vi "Auto_New.vi"() -> ()   [LabVIEW 2017]
uses:
  Control/Saurabh/prosucer_consumer_enum1.ctl
  Control/OUTPUT Cluster Indicator.ctl
  <vilib>/Utility/error.llb/DialogType.ctl
  <vilib>/addons/database/Connection.llb/DB Tools Open Connec (String).vi
  Global/DATA LOG.vi
  Global/Global 1.vi
  <vilib>/addons/database/NI_Database_API.lvlib
panel:
  out "SHIFT":string
  in  "BARCODE RECIPE":string(combo)
  out "PLC COM.":bool
  out "SHIFT_DATA":string[](array[string])
  out "stop":bool
  out "error out 2":errorcluster
  out "Shift 4":i32
  out "Time Stamp Out":timestamp[](array[timestamp]) format="%<%X>T"
  out "Time Stamp Out 4":timestamp[](array[timestamp]) format="%<%X>T"
  out "Shift_change":bool
  out "appended array":string[][](array[string])
  out "SHIFT_DATA 2":string[](array[string])
  in  "error in (no error)":errorcluster
  in  "Tab Control":T1(tab)
  out "OP 50":bool
  out "OP 40":bool
  out "OP 30":bool
  out "OP - 50":T2 {"RH Motor Screw" format="%#.2g N-m"; "LH Motor Screw" format="%#.2g N-m"; "Nut Torque" format="%#.2g N-m"}
  out "OP - 40":T3 {"Stack Load" format="%.2f kg"; "Dispalcement" format="%#.2g mm"; "LH Screw" format="%#.2g N-m"; "RH Screw" format="%#.2g N-m"}
  out "OP - 30":T4 {"Shaft Press Load" format="%#.2g kg"; "Displacement" format="%#.2g mm"}
  in  "stop 2":bool
  out "OP - 10":T5 {"Leak Rate" format="%#.2g SCCM"}
  in  "SIMULATE INPUT":bool[](array[boolean])=[FALSE, FALSE, FALSE, FALSE]
  out "OP - 20":T6 {"Top Load" format="%#.2g kg"; "Top Displace" format="%#.2g mm"; "Bottom Load" format="%#.2g kg"; "Bottom Displace" format="%#.2g mm"}
  out "OP 10 & 20":bool
  out "OP - 60":T7 {"Screw 6" format="%#.2g N-m"; "Screw 5" format="%#.2g N-m"; "Screw 4" format="%#.2g N-m"; "Screw 3" format="%#.2g N-m"; "Screw 2" format="%#.2g N-m"; "Screw 1" format="%#.2g N-m"}
  out "OP - 70":T8 {"Full Open" format="%#.4g V"; "Full Close" format="%#.4g V"}
  out "OP - 110":T9
  out "OP - 80":T10 {"Plug Press Load" format="%#.2f kg"}
  out "OP - 90":T11 {"Steam Leak" format="%#_g sccm"; "Seat Leak" format="%#_g LPM"}
  out "OP - 100":T12 {"Response Time REV" format="%#_g msec"; "Response time FWD" format="%#_g msec"; "Motor Full Open" format="%#.2f V"; "Motor Start Back" format="%#.2f V"; "Motor Full Close" format="%#.2f V"; "Motor Start Of Close" format="%#.2f V"; "Motor Peak" format="%#.2f A"; "Sensor O/P Full Close" format="%#.2f V"; "Sensor O/P Start Of Close" format="%#.2f V"; "Sensor O/P Open" format="%#.2f V"}
  out "OP 60":bool
  out "OP 70 & 80":bool
  out "OP 90 -100":bool
  out "OP 110":bool
  out "OP110 STATUS":dbl[](array[numeric])
  out "SCAN OP110":string[](array[string])
  out "OP100 STATUS":dbl[](array[numeric])
  out "SCAN OP100":string[](array[string])
  out "OP50 STATUS":dbl[](array[numeric])
  out "SCAN OP50":string[](array[string])
  out "OP90 STATUS":dbl[](array[numeric])
  out "SCAN OP90":string[](array[string])
  out "OP80 STATUS":dbl[](array[numeric])
  out "SCAN OP80":string[](array[string])
  out "OP70 STATUS":dbl[](array[numeric])
  out "SCAN OP70":string[](array[string])
  out "OP60 STATUS":dbl[](array[numeric])
  out "SCAN OP60":string[](array[string])
  out "OP40 STATUS":dbl[](array[numeric])
  out "SCAN OP40":string[](array[string])
  out "OP30 STATUS":dbl[](array[numeric])
  out "SCAN OP30":string[](array[string])
  out "OP20 STATUS":dbl[](array[numeric])
  out "SCAN OP20":string[](array[string])
  out "OP10 STATUS":dbl[](array[numeric])
  out "SCAN OP10":string[](array[string])
  out "resulting string":string
  out "PLC1 error":errorcluster
  out "PLC2 error":errorcluster
  out "PLC3 error":errorcluster
  out "PLC4 error":errorcluster
  out "PLC5 error":errorcluster
  out "PLC6 error":errorcluster
  out "PLC7 error":errorcluster
  out "PLC8 error":errorcluster
  # "Op10 20\nOp30\nOp 40\nOp50\nOp60\nOp70-80\nOp 90-100-110"
  # "SENSOR MIN VLTG"
  # "OP - 50"
  # "OP - 40"
  # "OP - 30"
  # "OP - 10"
  # "OP - 20"
  # "OP - 60"
  # "OP - 70"
  # "OP - 110"
  # "OP - 80"
  # "OP - 90"
  # "OP - 100"
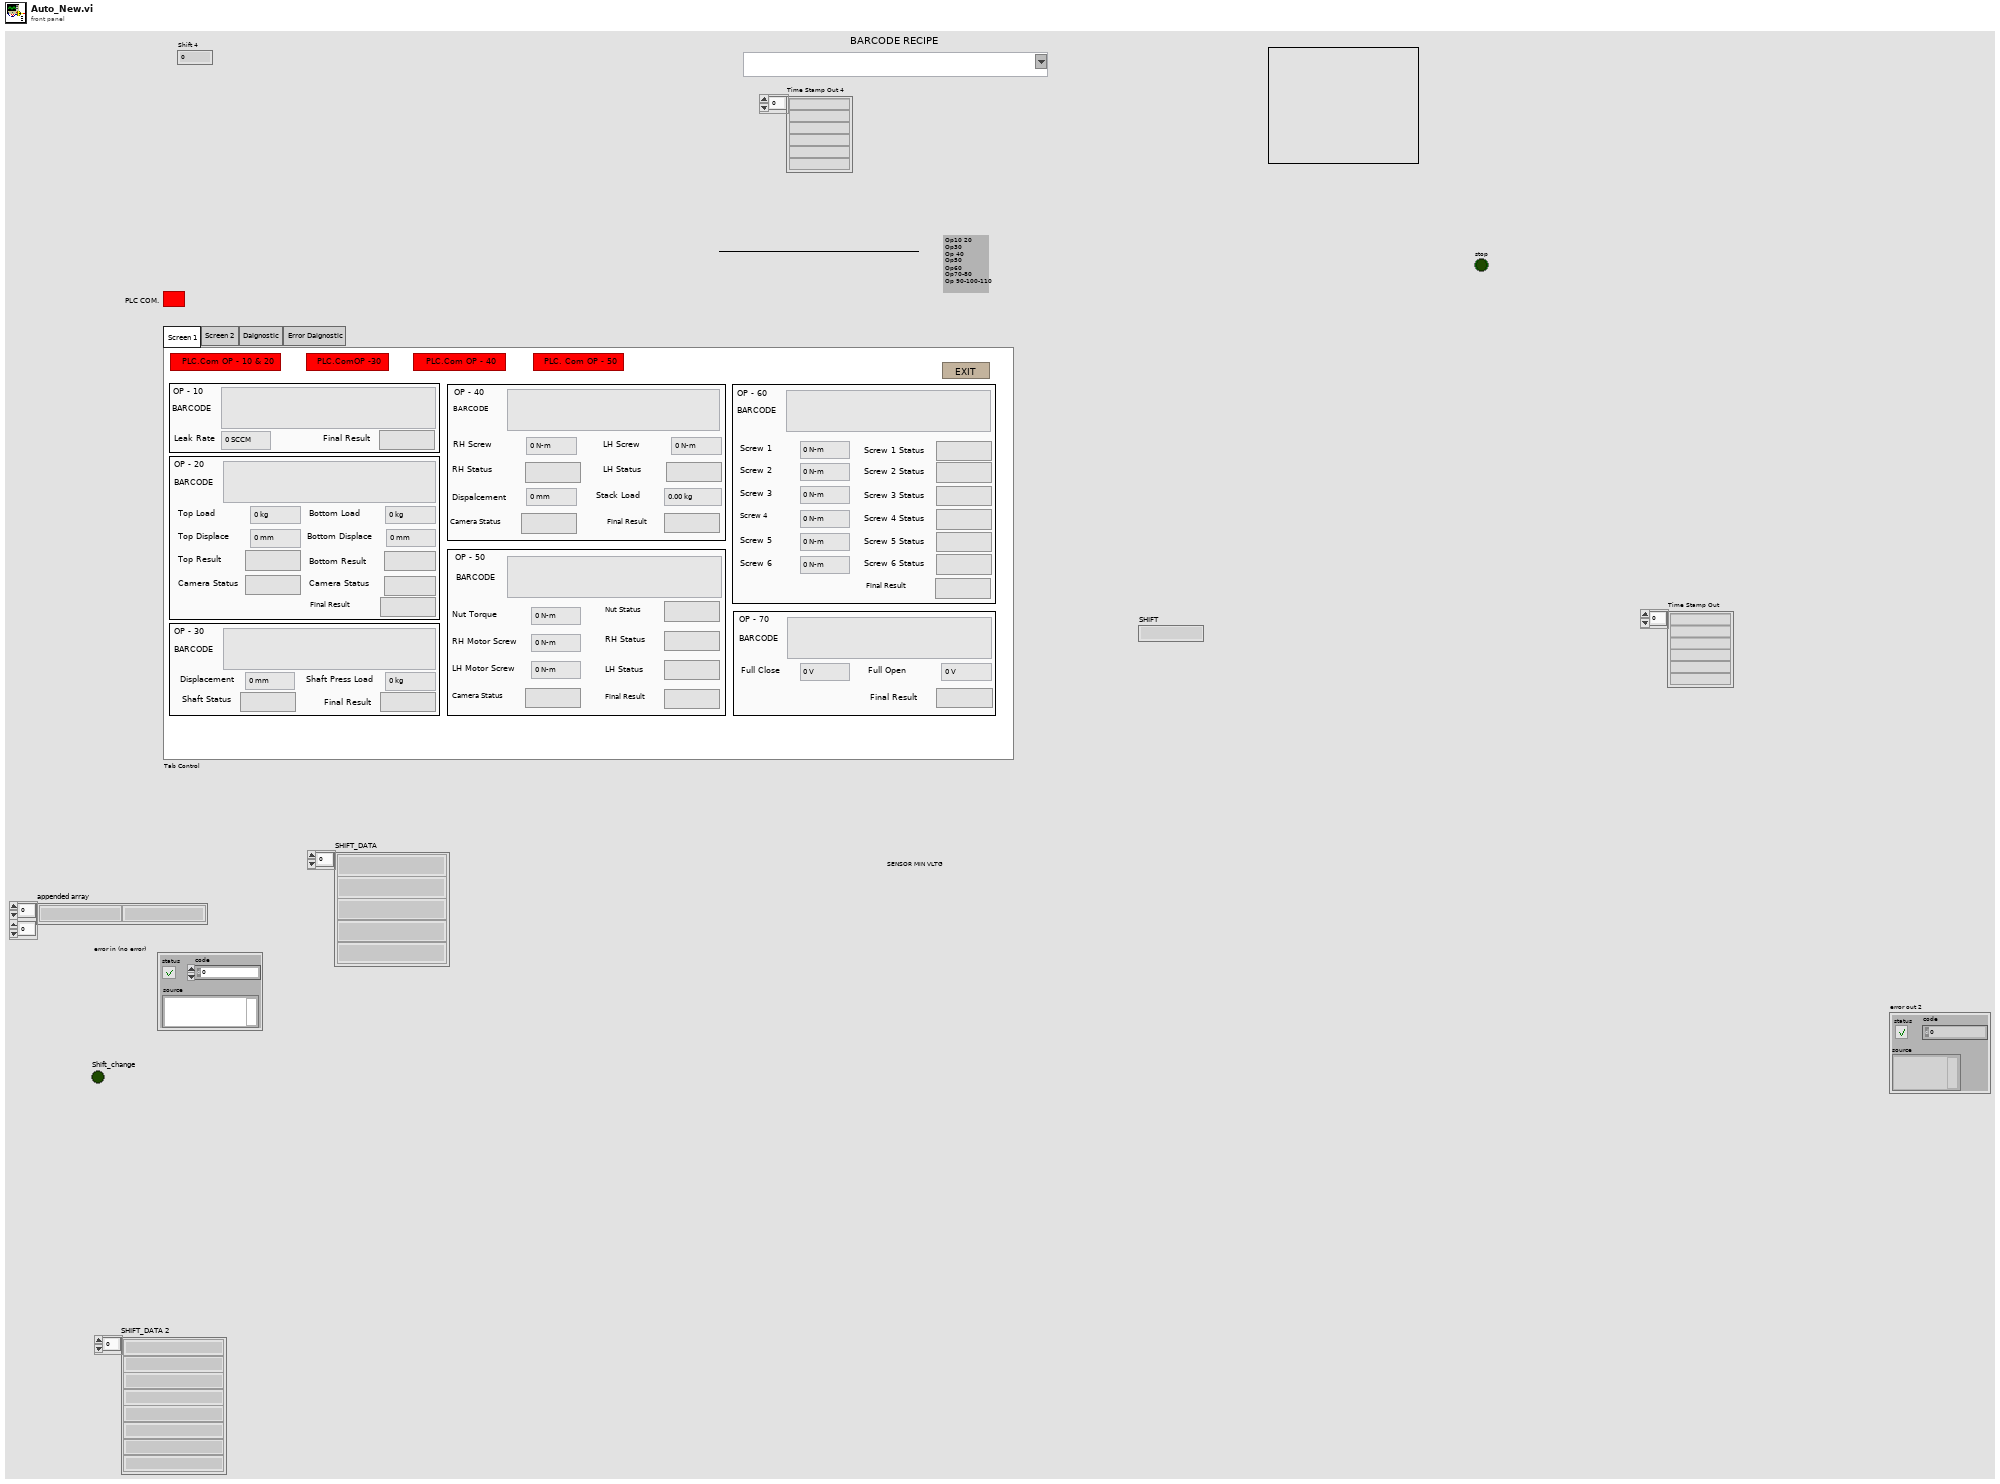
[diagram p1: front panel]
types:
  T1 = enum32{"Screen 1", "Screen 2", "Daignostic", "Error Daignostic"}
  T2 = cluster{"BARCODE":string, "Nut Torque":dbl, "LH Motor Screw":dbl, "LH Status":bool, "RH Status":bool, "RH Motor Screw":dbl, "Final Result":bool, "Nut Status":bool, "Camera Status":bool}
  T3 = cluster{"BARCODE":string, "RH Screw":dbl, "LH Screw ":dbl, "RH Status":bool, "LH Status":bool, "Dispalcement ":dbl, "Stack Load ":dbl, "Final Result":bool, "Camera Status":bool}
  T4 = cluster{"BARCODE":string, "Displacement":dbl, "Shaft Press Load":dbl, "Shaft Status":bool, "Final Result":bool}
  T5 = cluster{"BARCODE":string, "Leak Rate":dbl, "Final Result":bool}
  T6 = cluster{"BARCODE":string, "Bottom Displace":dbl, "Bottom Load":dbl, "Camera Status":bool, "Bottom Result":bool, "Top Displace":dbl, "Top Load ":dbl, "Camera Status":bool, "Top Result":bool, "Final Result":bool}
  T7 = cluster{"BARCODE":string, "Screw 1":dbl, "Screw 2":dbl, "Screw 1 Status":bool, "Screw 2 Status":bool, "Screw 3":dbl, "Final Result":bool, "Screw 3 Status":bool, "Screw 4":dbl, "Screw 5":dbl, "Screw 4 Status":bool, "Screw 5 Status":bool, "Screw 6":dbl, "Screw 6 Status":bool}
  T8 = cluster{"BARCODE":string, "Full Close":dbl, "Full Open":dbl, "Final Result":bool}
  T9 = cluster{"BARCODE":string, "BIN\nNumber":string, "PALLET\nNumber":string}
  T10 = cluster{"BARCODE":string, "Plug Press Load":dbl, "Final Result":bool, "Loctite Status":bool}
  T11 = cluster{"BARCODE":string, "Seat Leak":dbl, "Seat Status":bool, "Steam Leak":dbl, "Final Result":bool}
  T12 = cluster{"BARCODE":string, "Sensor O/P Open":dbl, "Sensor O/P Start Of Close":dbl, "Final Result":bool, "Sensor O/P Full Close":dbl, "Motor Peak":dbl, "Motor Start Of Close":dbl, "Motor Full Close":dbl, "Motor Start Back":dbl, "Motor Full Open":dbl, "Response time FWD":dbl, "Response Time REV":dbl, "Camera Status":bool}
  T13 = typedef "OUTPUT Cluster Indicator.ctl" = cluster{"OP - 10":cluster{"BARCODE":string, "LEAK RATE":dbl, "RESULT":bool}, "OP - 30":cluster{"BARCODE":string, "Displacement":dbl, "Load":dbl, "Middle Gear Shaft Status":bool, "Final Result":bool}, "OP - 60":cluster{"BARCODE":string, "Screw 1 Data":dbl, "Screw 2 data":dbl, "Screw 1 Status":bool, "Screw 2 Status":bool, "Screw3 Data":dbl, "Final Result":bool, "Screw3 Status":bool, "Screw4 Data":dbl, "Screw5 Data":dbl, "Screw4 Status":bool, "Screw5 Status":bool, "Screw6 Data":dbl, "Screw6 Status":bool}, "OP - 70":cluster{"BARCODE":string, "Sensor MIN Vltg":dbl, "Sensor MAX Vltg":dbl, "Final Result":bool}, "OP - 80":cluster{"BARCODE":string, "Load":dbl, "Final Result":bool, "Dispensing":bool}, "OP - 90":cluster{"BARCODE":string, "Seat LT Data":dbl, "Seat Status":bool, "Steam LT Data":dbl, "Final Result":bool}, "OP - 110":cluster{"BARCODE":string, "BIN\nNumber":string, "PALLET\nNumber":string}, "OP - 20":cluster{"BARCODE":string, "Bottom Displace":dbl, "Bottom Load":dbl, "Camera Status":bool, "Bottom Result":bool, "Top Displace":dbl, "Top Load ":dbl, "Camera Status":bool, "Top Result":bool, "Final Result":bool}, "OP - 50":cluster{"BARCODE":string, "Nut Torque":dbl, "LH Motor Screw":dbl, "LH Status":bool, "RH Status":bool, "RH Motor Screw":dbl, "Final Result":bool, "Nut Status":bool, "Camera Status":bool}, "OP - 100":cluster{"BARCODE":string, "Sensor O/P Open":dbl, "Sensor O/P Start Of Close":dbl, "Final Result":bool, "Sensor O/P Full Close":dbl, "Motor Peak":dbl, "Motor Start Of Close":dbl, "Motor Full Close":dbl, "Motor Start Back":dbl, "Motor Full Open":dbl, "Response time FWD":dbl, "Response Time REV":dbl, "Camera Status":bool}, "OP - 40":cluster{"BARCODE":string, "RH Screw":dbl, "LH Screw ":dbl, "RH Status":bool, "LH Status":bool, "Dispalcement ":dbl, "Stack Load ":dbl, "Final Result":bool, "Camera Status":bool}}
  T14 = cluster{"OP - 10":cluster{"BARCODE":string, "LEAK RATE":dbl, "RESULT":bool}, "OP - 30":cluster{"BARCODE":string, "Displacement":dbl, "Load":dbl, "Middle Gear Shaft Status":bool, "Final Result":bool}, "OP - 60":cluster{"BARCODE":string, "Screw 1 Data":dbl, "Screw 2 data":dbl, "Screw 1 Status":bool, "Screw 2 Status":bool, "Screw3 Data":dbl, "Final Result":bool, "Screw3 Status":bool, "Screw4 Data":dbl, "Screw5 Data":dbl, "Screw4 Status":bool, "Screw5 Status":bool, "Screw6 Data":dbl, "Screw6 Status":bool}, "OP - 70":cluster{"BARCODE":string, "Sensor MIN Vltg":dbl, "Sensor MAX Vltg":dbl, "Final Result":bool}, "OP - 80":cluster{"BARCODE":string, "Load":dbl, "Final Result":bool, "Dispensing":bool}, "OP - 90":cluster{"BARCODE":string, "Seat LT Data":dbl, "Seat Status":bool, "Steam LT Data":dbl, "Final Result":bool}, "OP - 110":cluster{"BARCODE":string}, "OP - 20":cluster{"BARCODE":string, "Bottom Displace":dbl, "Bottom Load":dbl, "Camera Status":bool, "Bottom Result":bool, "Top Displace":dbl, "Top Load ":dbl, "Camera Status":bool, "Top Result":bool, "Final Result":bool}, "OP - 40":cluster{"BARCODE":string, "RH Screw":dbl, "LH Screw ":dbl, "RH Status":bool, "LH Status":bool, "Dispalcement ":dbl, "Stack Load ":dbl, "Final Result":bool}, "OP - 50":cluster{"BARCODE":string, "Nut Torque":dbl, "LH Motor Screw":dbl, "LH Status":bool, "RH Status":bool, "RH Motor Screw":dbl, "Final Result":bool, "Nut Status":bool, "Camera Status":bool}, "OP - 100":cluster{"BARCODE":string, "Sensor O/P Open":dbl, "Sensor O/P Start Of Close":dbl, "Final Result":bool, "Sensor O/P Full Close":dbl, "Motor Peak":dbl, "Motor Start Of Close":dbl, "Motor Full Close":dbl, "Motor Start Back":dbl, "Motor Full Open":dbl, "Response time FWD":dbl, "Response Time REV":dbl, "Camera Status":bool}}
  T15 = typedef "prosucer_consumer_enum1.ctl" = enum16{"-1", "SCAN1", "SCAN2", "SCAN3", "SCAN4", "SCAN5", "SCAN6", "SCAN7", "SCAN8", "SCAN9", "SCAN10", "SCAN11", "STOP", "DATALOG1", "DATALOG2", "DATALOG3", "DATALOG4", "DATALOG5", "DATALOG6", "DATALOG7", "DATALOG8", "DATALOG9", "DATALOG10", "DATALOG11", "CYCLE_START1", "CYCLE_START2", "CYCLE_START3", "CYCLE_START4", "BARCODE RECIPE", "EMERGENCY STOP"}
  T16 = typedef "NI_Database_API.lvlib/Conn ObjectReference.ctl" = refnum<k1>
  T17 = typedef "DialogType.ctl" = u16
  T18 = cluster{"trimmed string":string, "SHIFT":string, "date/time string":string, string, "Input 2":string}
  T19 = cluster{"SHIFT":string, "date/time string":string, "Input 2":string, string}
  T20 = cluster{"date/time string":string, "Input 2":string, "Input 2":string, "Input 2":string, "Input 2":string, "Input 2":string, "Input 2":string, "Input 2":string, "Input 2":string, "Input 2":string, "Input 2":string}
  T21 = cluster{"date/time string":string, "SHIFT":string, "Input 2":string, "Input 2":string, "Input 2":string, "Input 2":string, "Input 2":string, "Input 2":string, "Input 2":string, "Input 2":string, "Input 2":string, "Input 2":string}
  T22 = cluster{"date/time string":string, "Input 2":string, "Input 2":string, "Input 2":string, "Input 2":string}
  T23 = cluster{"date/time string":string, "SHIFT":string, "Input 2":string, "Input 2":string, "Input 2":string, "Input 2":string}
  T24 = cluster{"date/time string":string, "Input 2":string, "Input 2":string, "Input 2":string, "Input 2":string, "Input 2":string, "Input 2":string, "Input 2":string, "Input 2":string}
  T25 = cluster{"date/time string":string, "SHIFT":string, "Input 2":string, "Input 2":string, "Input 2":string, "Input 2":string, "Input 2":string, "Input 2":string, "Input 2":string, "Input 2":string}
  T26 = cluster{"date/time string":string, "SHIFT":string, "Input 2":string, "Input 2":string, "Input 2":string, "Input 2":string, "Input 2":string, "Input 2":string}
  T27 = cluster{"date/time string":string, "Input 2":string, "Input 2":string, "Input 2":string, "Input 2":string, "Input 2":string, "Input 2":string, "Input 2":string, "Input 2":string, "Input 2":string, "Input 2":string, "Input 2":string, "Input 2":string, "Input 2":string}
  T28 = cluster{"date/time string":string, "SHIFT":string, "Input 2":string, "Input 2":string, "Input 2":string, "Input 2":string, "Input 2":string, "Input 2":string, "Input 2":string, "Input 2":string, "Input 2":string, "Input 2":string, "Input 2":string, "Input 2":string}
  T29 = cluster{"date/time string":string, "Input 2":string, "Input 2":string, "Input 2":string}
  T30 = cluster{"date/time string":string, "SHIFT":string, "Input 2":string, "Input 2":string, "Input 2":string}
  T31 = cluster{"Input 2":string, "SHIFT":string, "date/time string":string, "Input 2":string, "Input 2":string, "Input 2":string}
  T32 = cluster{"date/time string":string, "trimmed string":string, "trimmed string":string}
  T33 = cluster{"BARCODE":string, "Seat LT Data":dbl, "Seat Status":bool, "Steam LT Data":dbl, "Final Result":bool}
  T34 = cluster{"BARCODE":string, "LEAK RATE":dbl, "RESULT":bool}
  T35 = cluster{"BARCODE":string, "Displacement":dbl, "Load":dbl, "Middle Gear Shaft Status":bool, "Final Result":bool}
  T36 = cluster{"BARCODE":string, "Screw 1 Data":dbl, "Screw 2 data":dbl, "Screw 1 Status":bool, "Screw 2 Status":bool, "Screw3 Data":dbl, "Final Result":bool, "Screw3 Status":bool, "Screw4 Data":dbl, "Screw5 Data":dbl, "Screw4 Status":bool, "Screw5 Status":bool, "Screw6 Data":dbl, "Screw6 Status":bool}
  T37 = cluster{"BARCODE":string, "Sensor MIN Vltg":dbl, "Sensor MAX Vltg":dbl, "Final Result":bool}
  T38 = cluster{"BARCODE":string, "Load":dbl, "Final Result":bool, "Dispensing":bool}
  T39 = enum32{"invalid app kind", "Development System", "Run Time System", "Student Edition", "Embedded LabVIEW", "Evaluation", "Custom"}
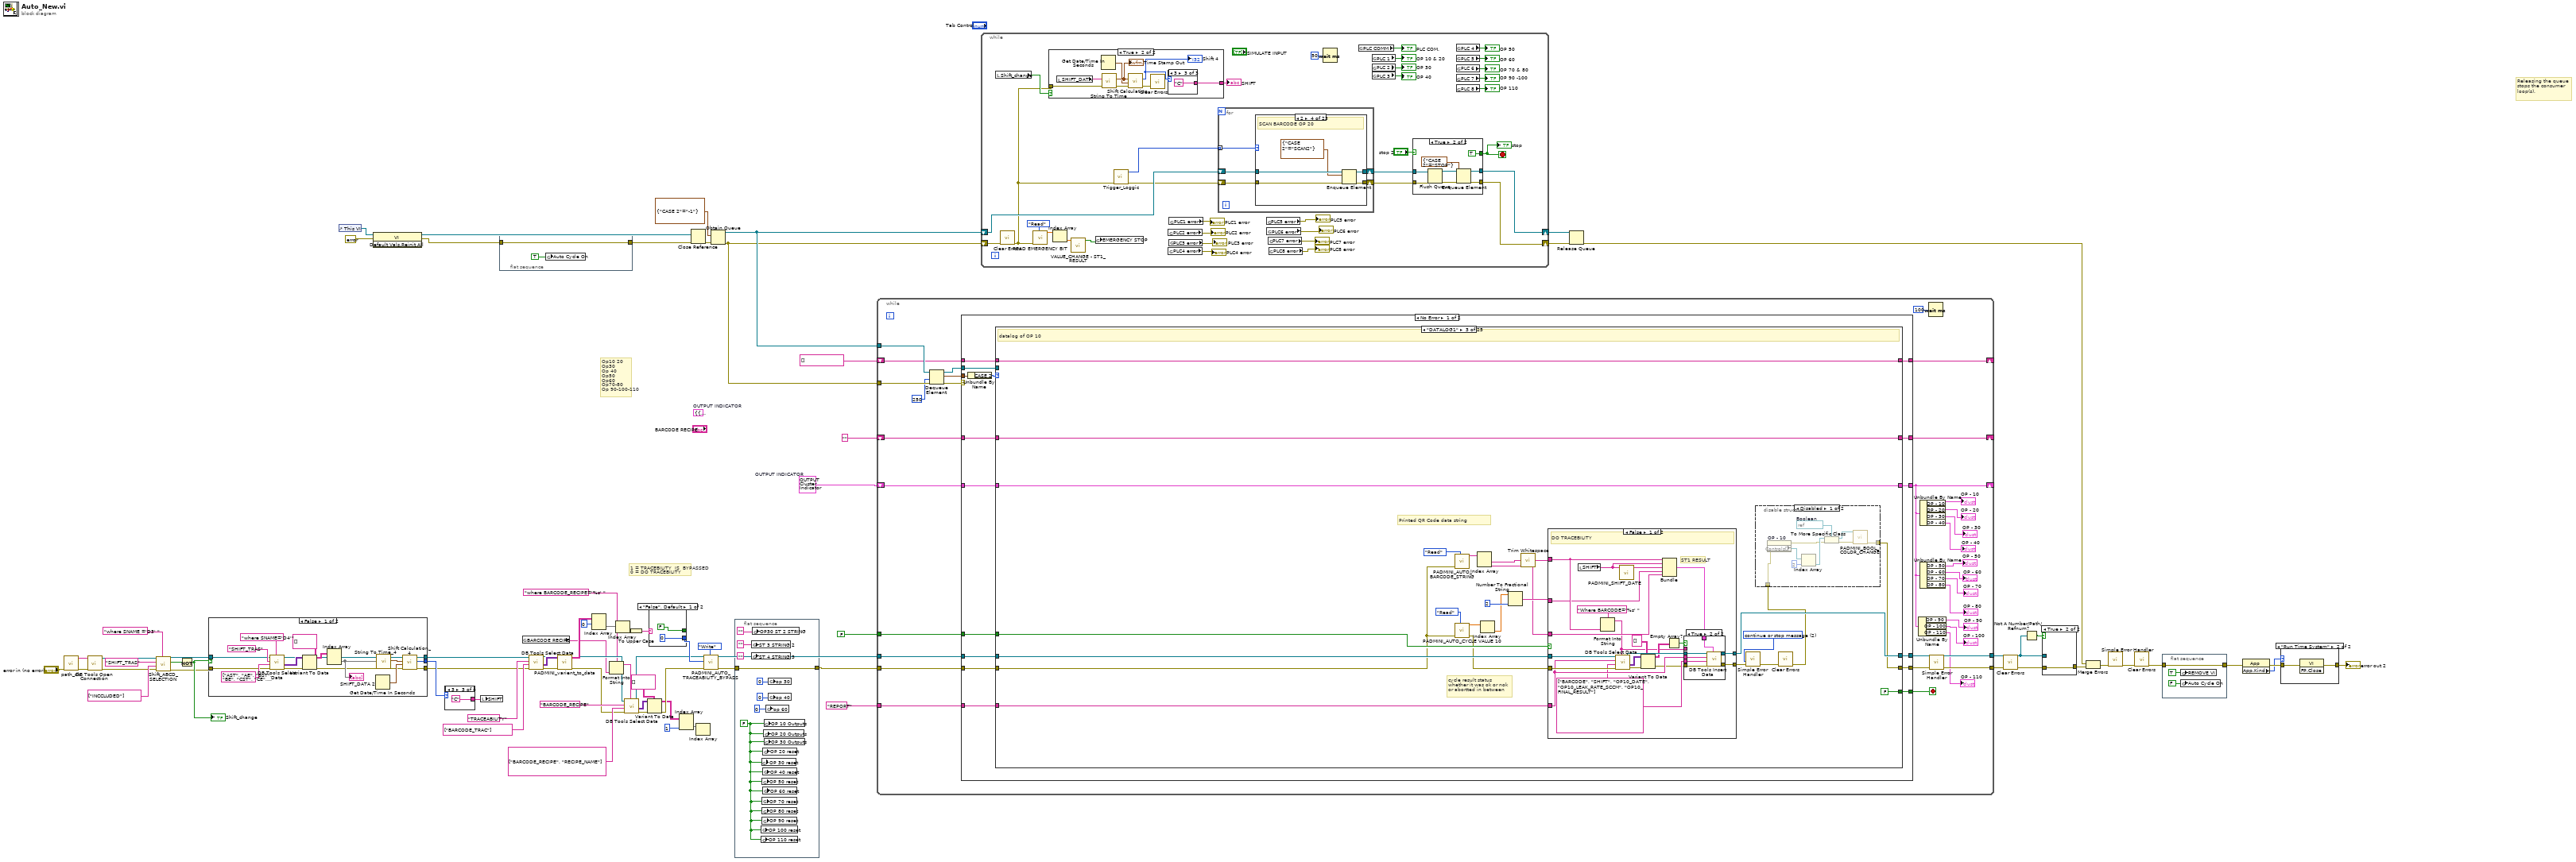
[diagram p0: block diagram]
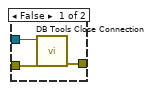
[diagram p2: hidden frame]
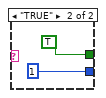
[diagram p3: hidden frame]
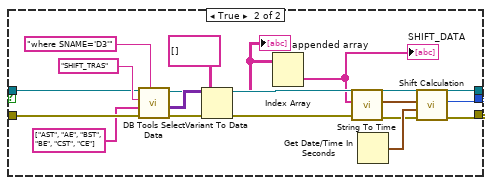
[diagram p4: hidden frame]
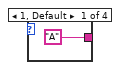
[diagram p5: hidden frame]
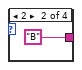
[diagram p6: hidden frame]
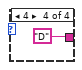
[diagram p7: hidden frame]
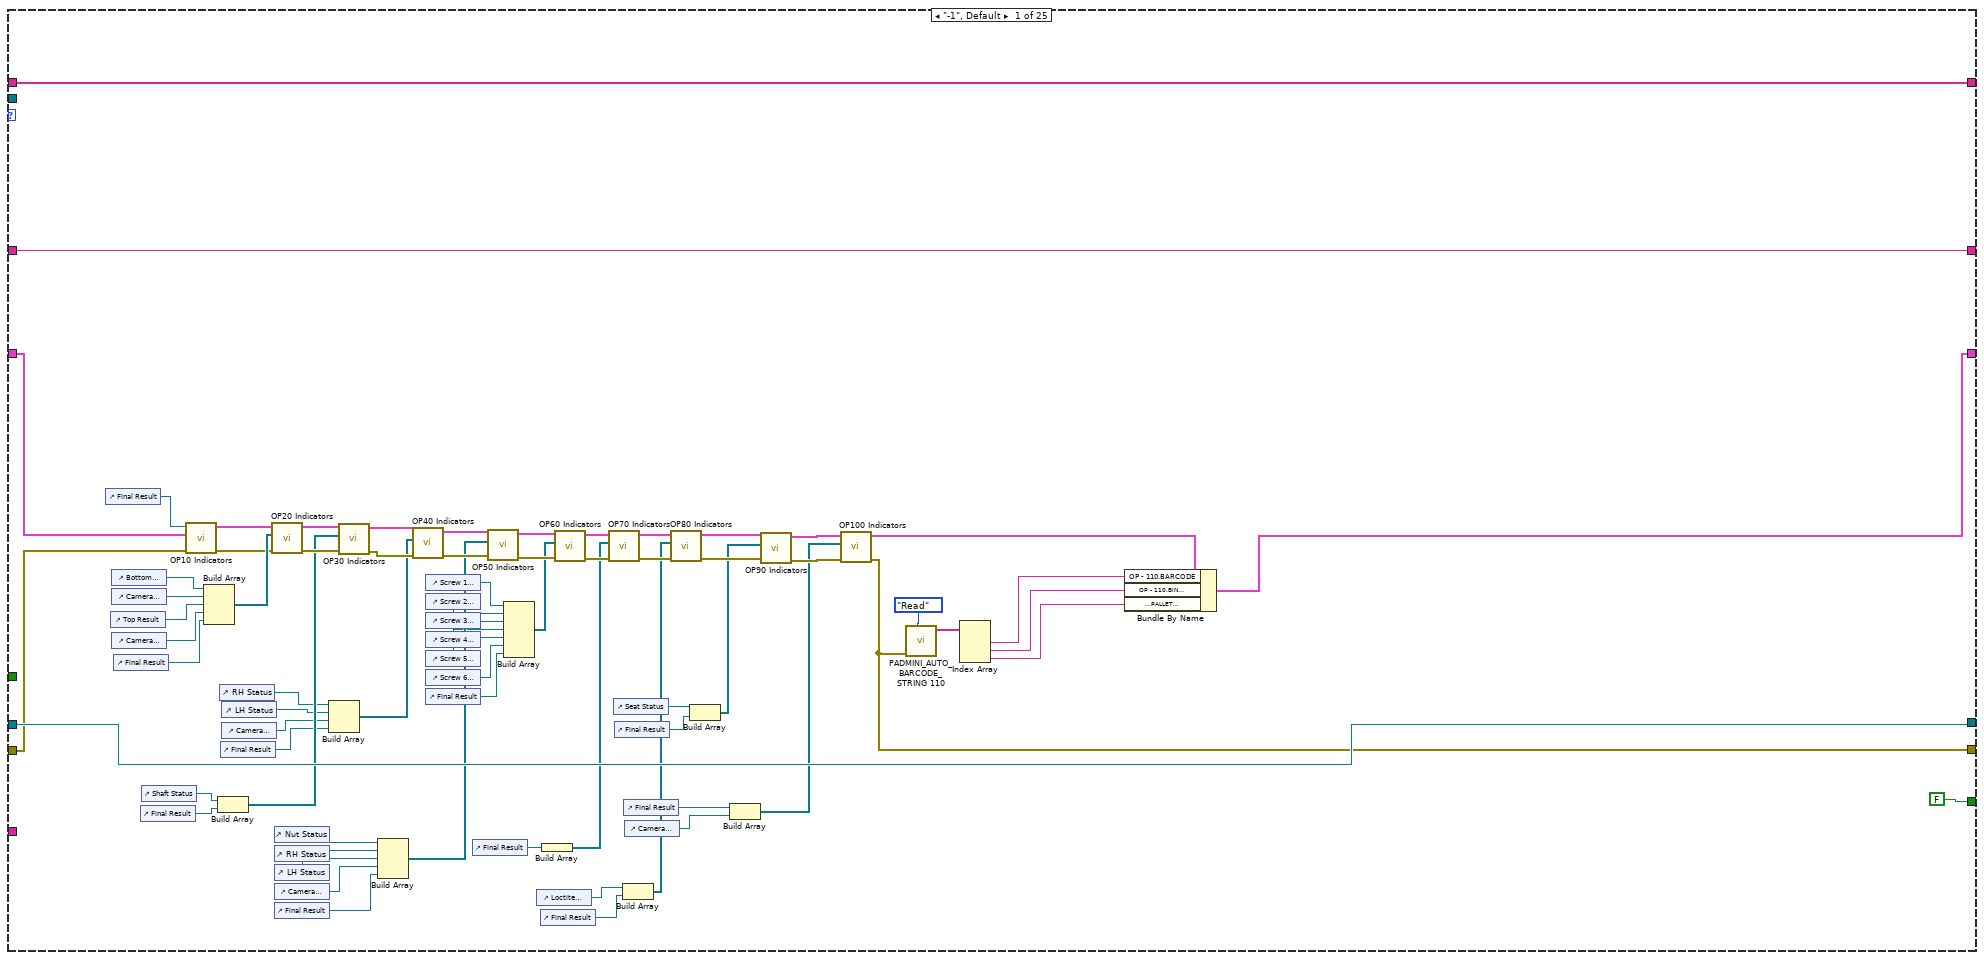
[diagram p8: hidden frame]
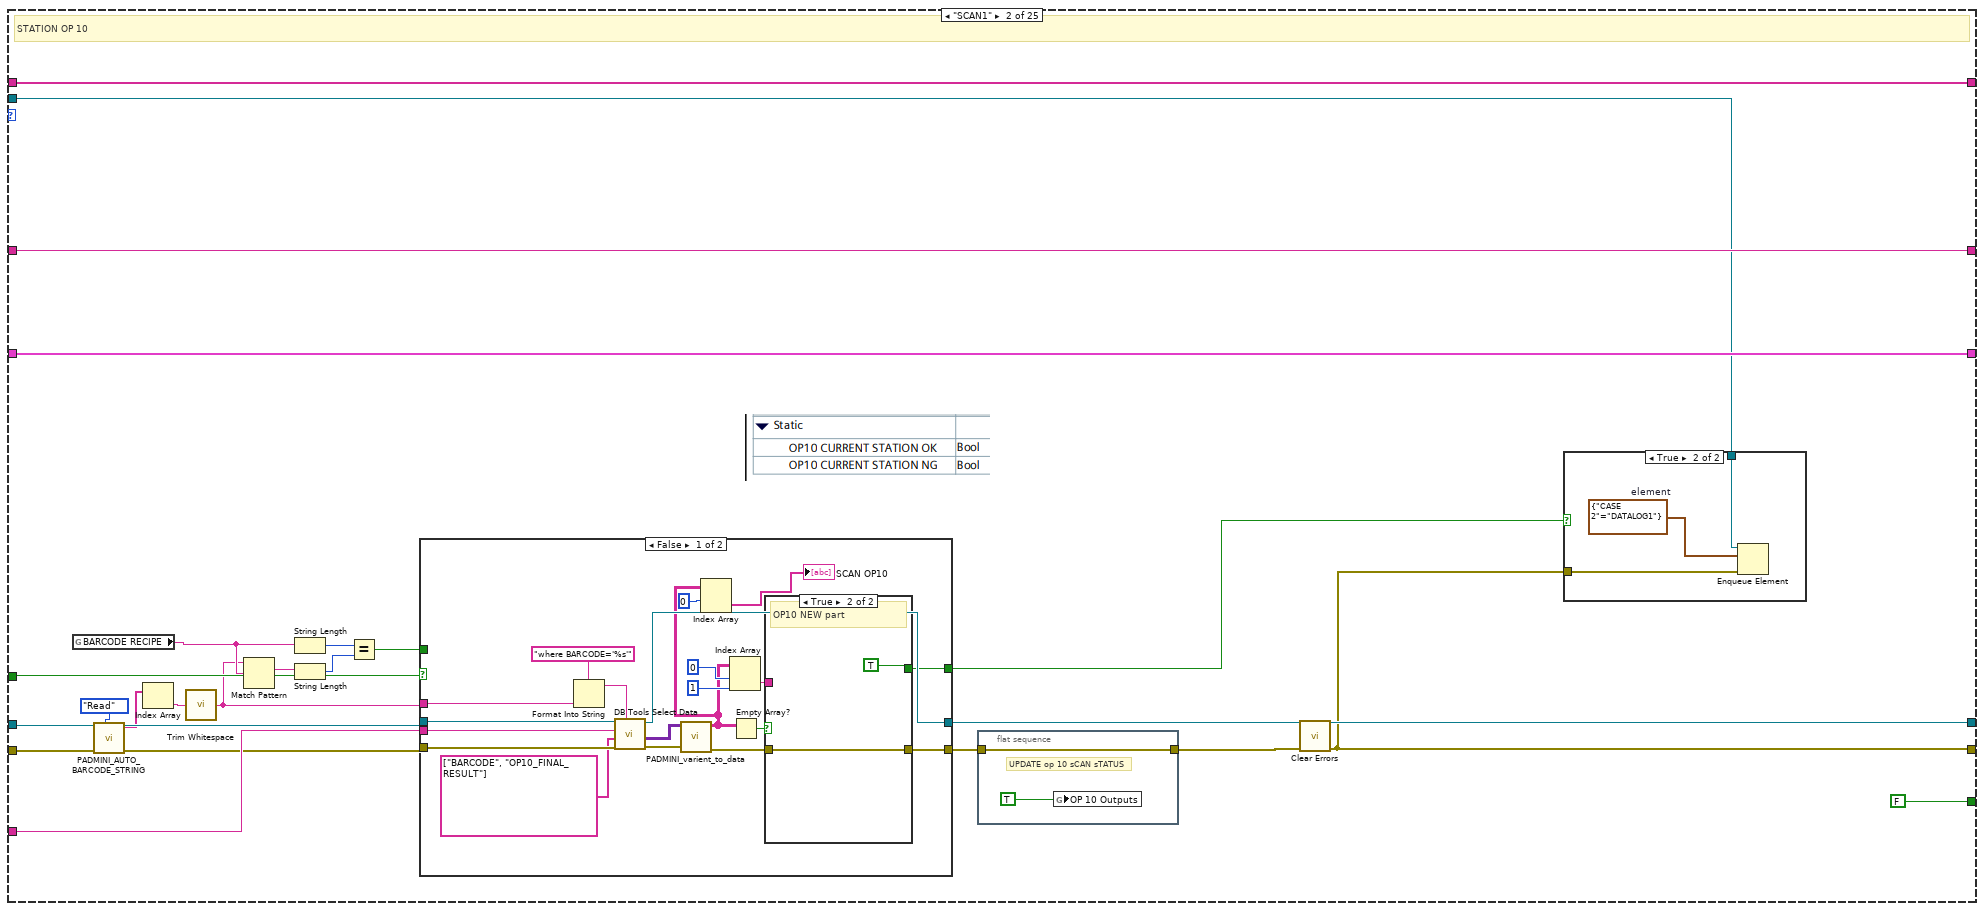
[diagram p9: hidden frame]
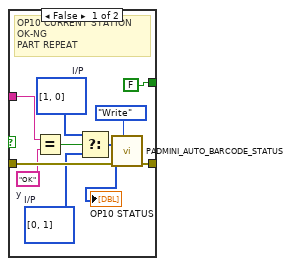
[diagram p11: hidden frame]
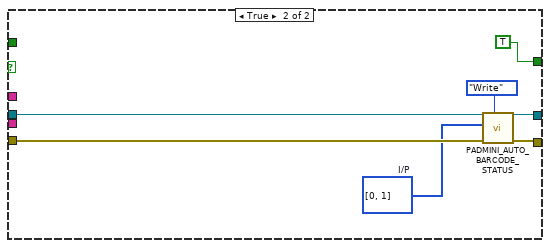
[diagram p12: hidden frame]
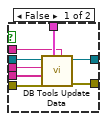
[diagram p14: hidden frame]
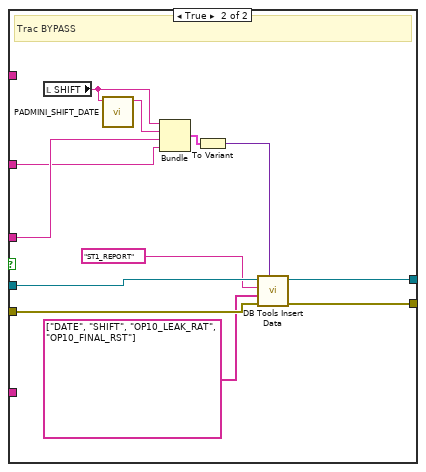
[diagram p15: hidden frame]
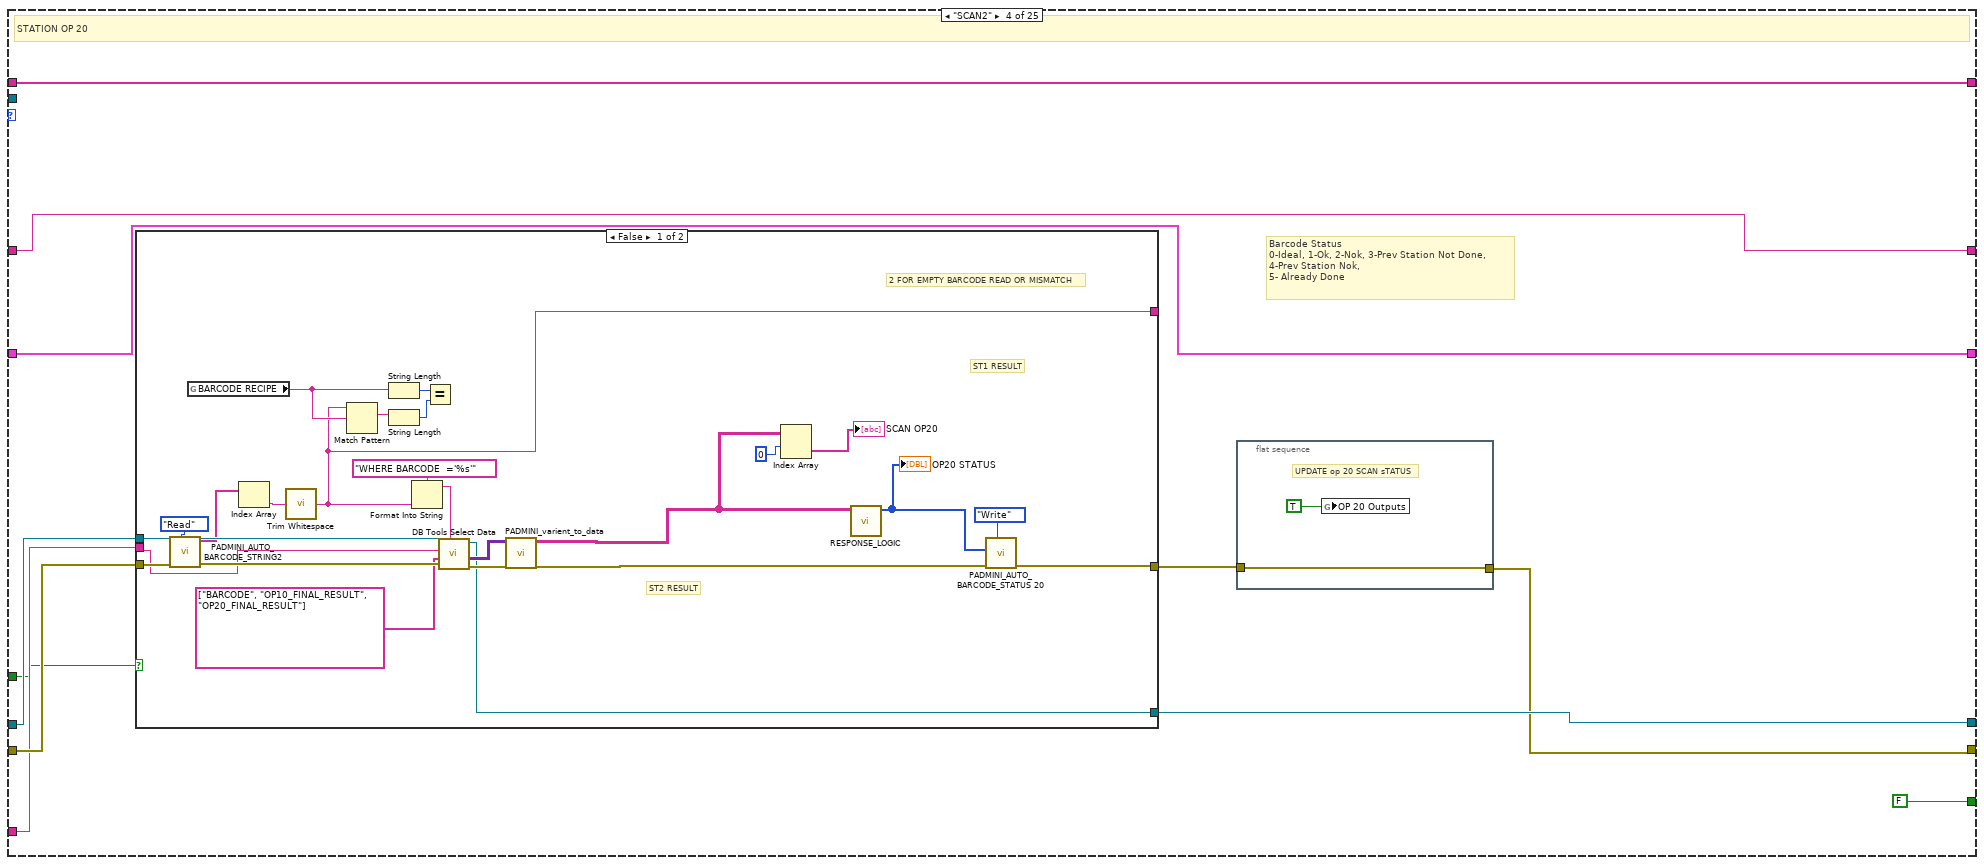
[diagram p16: hidden frame]
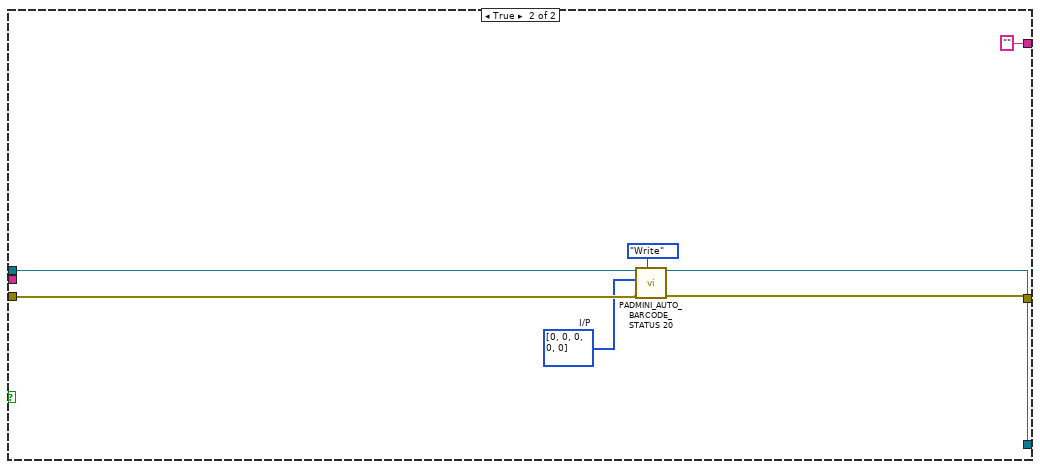
[diagram p17: hidden frame]
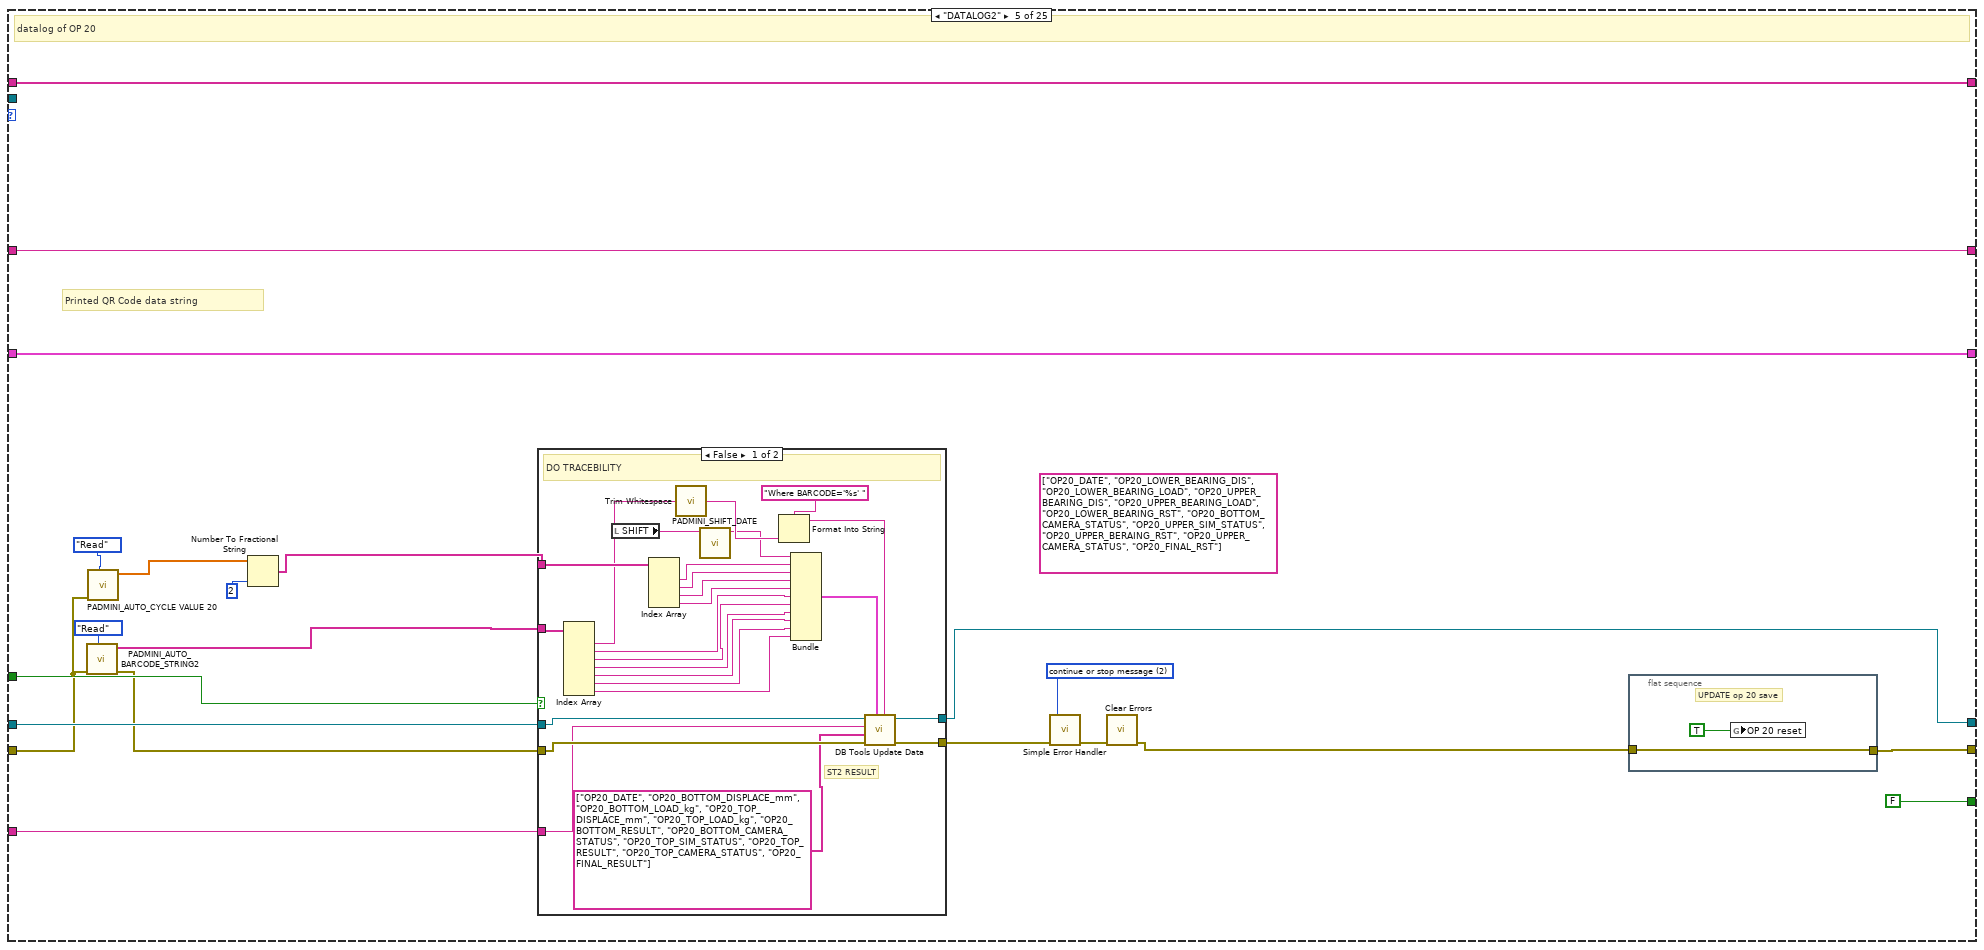
[diagram p18: hidden frame]
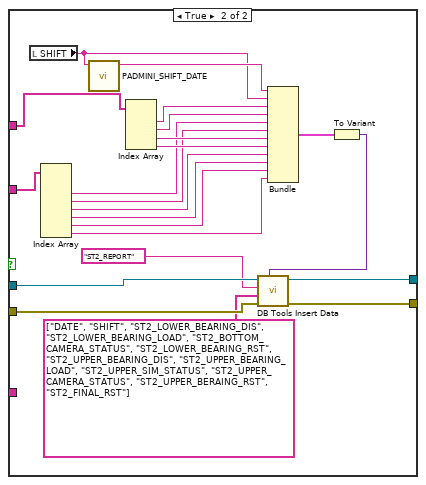
[diagram p19: hidden frame]
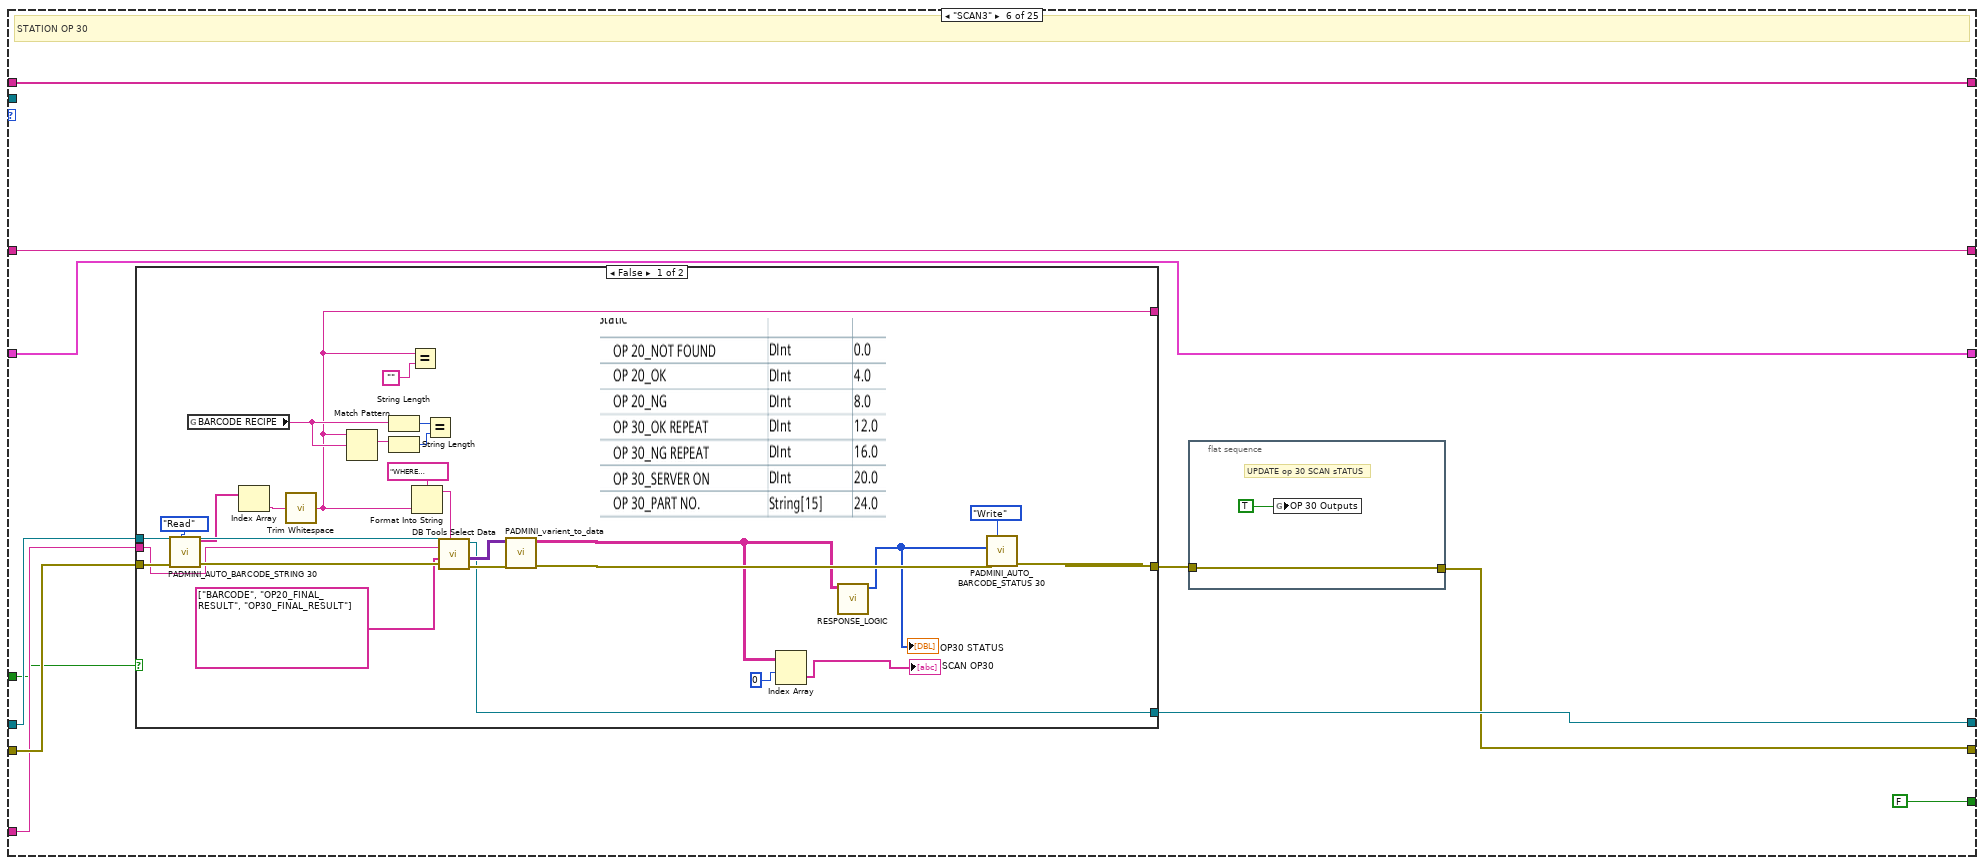
[diagram p20: hidden frame]
diagram:
  w3 = T13 {"OP - 10"={"BARCODE"="", "LEAK RATE"=0.0, "RESULT"=FALSE}, "OP - 30"={"BARCODE"="", "Displacement"=0.0, "Load"=0.0, "Middle Gear Shaft Status"=FALSE, "Final Result"=FALSE}, "OP - 60"={"BARCODE"="", "Screw 1 Data"=0.0, "Screw 2 data"=0.0, "Screw 1 Status"=FALSE, "Screw 2 Status"=FALSE, "Screw3 Data"=0.0, "Final Result"=FALSE, "Screw3 Status"=FALSE, "Screw4 Data"=0.0, "Screw5 Data"=0.0, "Screw4 Status"=FALSE, "Screw5 Status"=FALSE, "Screw6 Data"=0.0, "Screw6 Status"=FALSE}, "OP - 70"={"BARCODE"="", "Sensor MIN Vltg"=0.0, "Sensor MAX Vltg"=0.0, "Final Result"=FALSE}, "OP - 80"={"BARCODE"="", "Load"=0.0, "Final Result"=FALSE, "Dispensing"=FALSE}, "OP - 90"={"BARCODE"="", "Seat LT Data"=0.0, "Seat Status"=FALSE, "Steam LT Data"=0.0, "Final Result"=FALSE}, "OP - 110"={"BARCODE"="", "BIN\nNumber"="", "PALLET\nNumber"=""}, "OP - 20"={"BARCODE"="", "Bottom Displace"=0.0, "Bottom Load"=0.0, "Camera Status"=FALSE, "Bottom Result"=TRUE, "Top Displace"=0.0, "Top Load "=0.0, "Camera Status"=FALSE, "Top Result"=FALSE, "Final Result"=FALSE}, "OP - 50"={"BARCODE"="", "Nut Torque"=0.0, "LH Motor Screw"=0.0, "LH Status"=FALSE, "RH Status"=FALSE, "RH Motor Screw"=0.0, "Final Result"=FALSE, "Nut Status"=FALSE, "Camera Status"=FALSE}, "OP - 100"={"BARCODE"="", "Sensor O/P Open"=0.0, "Sensor O/P Start Of Close"=0.0, "Final Result"=FALSE, "Sensor O/P Full Close"=0.0, "Motor Peak"=0.0, "Motor Start Of Close"=0.0, "Motor Full Close"=0.0, "Motor Start Back"=0.0, "Motor Full Open"=0.0, "Response time FWD"=0.0, "Response Time REV"=0.0, "Camera Status"=FALSE}, "OP - 40"={"BARCODE"="", "RH Screw"=0.0, "LH Screw "=0.0, "RH Status"=FALSE, "LH Status"=FALSE, "Dispalcement "=0.0, "Stack Load "=0.0, "Final Result"=FALSE, "Camera Status"=TRUE}}  # OUTPUT INDICATOR
  (unwired) T14 {"OP - 10"={"BARCODE"="", "LEAK RATE"=0.0, "RESULT"=FALSE}, "OP - 30"={"BARCODE"="", "Displacement"=0.0, "Load"=0.0, "Middle Gear Shaft Status"=FALSE, "Final Result"=FALSE}, "OP - 60"={"BARCODE"="", "Screw 1 Data"=0.0, "Screw 2 data"=0.0, "Screw 1 Status"=FALSE, "Screw 2 Status"=FALSE, "Screw3 Data"=0.0, "Final Result"=FALSE, "Screw3 Status"=FALSE, "Screw4 Data"=0.0, "Screw5 Data"=0.0, "Screw4 Status"=FALSE, "Screw5 Status"=FALSE, "Screw6 Data"=0.0, "Screw6 Status"=FALSE}, "OP - 70"={"BARCODE"="", "Sensor MIN Vltg"=0.0, "Sensor MAX Vltg"=0.0, "Final Result"=FALSE}, "OP - 80"={"BARCODE"="", "Load"=0.0, "Final Result"=FALSE, "Dispensing"=FALSE}, "OP - 90"={"BARCODE"="", "Seat LT Data"=0.0, "Seat Status"=FALSE, "Steam LT Data"=0.0, "Final Result"=FALSE}, "OP - 110"={"BARCODE"=""}, "OP - 20"={"BARCODE"="", "Bottom Displace"=0.0, "Bottom Load"=0.0, "Camera Status"=FALSE, "Bottom Result"=TRUE, "Top Displace"=0.0, "Top Load "=0.0, "Camera Status"=FALSE, "Top Result"=FALSE, "Final Result"=FALSE}, "OP - 40"={"BARCODE"="", "RH Screw"=0.0, "LH Screw "=0.0, "RH Status"=FALSE, "LH Status"=FALSE, "Dispalcement "=0.0, "Stack Load "=0.0, "Final Result"=FALSE}, "OP - 50"={"BARCODE"="", "Nut Torque"=0.0, "LH Motor Screw"=0.0, "LH Status"=FALSE, "RH Status"=FALSE, "RH Motor Screw"=0.0, "Final Result"=FALSE, "Nut Status"=FALSE, "Camera Status"=FALSE}, "OP - 100"={"BARCODE"="", "Sensor O/P Open"=0.0, "Sensor O/P Start Of Close"=0.0, "Final Result"=FALSE, "Sensor O/P Full Close"=0.0, "Motor Peak"=0.0, "Motor Start Of Close"=0.0, "Motor Full Close"=0.0, "Motor Start Back"=0.0, "Motor Full Open"=0.0, "Response time FWD"=0.0, "Response Time REV"=0.0, "Camera Status"=FALSE}}  # OUTPUT INDICATOR
  # "Op10 20\nOp30\nOp 40\nOp50\nOp60\nOp70-80\nOp 90-100-110"
  # "1 = TRACEBILITY  IS  BYPASSED\n0 = DO TRACEBILITY"
  # "Releasing the queue stops the consumer loop(s)."
  n1 = call "path_db.vi"("error in"="error in (no error)") -> ("error out"=w50:errorcluster, "resulting string"=w70:string)  [unwired: 9 in]
  n2 = call-poly <vilib>:"DB Tools Open Connection.vi"("error in (no error)"=w50, "connection information"=w70) -> ("error out"=w49:errorcluster, "connection reference"=w43:T16)  [unwired: 6 in]
  n3 = call "Shift_ABCD_SELECTION.vi"("Where"="where SNAME ='D3' ", "error in (no error)"=w49, "Array"=string[] ["INCCLUDED"], "table"="SHIFT_TRAS", "Refnum in"=w43) -> ("error out"=w7:errorcluster, "Boolean"=w62:bool, "Refnum out"=w63:T16)  [unwired: 4 in]
  n4 = Not(x=w62) -> (.not. x?=w61:bool)
  "Shift_change" <- w61
  n5 = case shown="False" w61 {
    tunnel: [w75 w99] -> w67
    tunnel: w63 -> [w78 w97]
    tunnel: w7 -> [w77 w96]
    tunnel: [w76 w95] -> w32
    tunnel: [w74 w89] -> w31
    frame False {
      n6 = call <vilib>:"DB Tools Select Data.vi"("condition"="where SNAME='D4'", "error in (no error)"=w77, "columns"=string[] ["AST", "AE", "BST", "BE", "CST", "CE", "DST", "DE"], "table"="SHIFT_TRAS", "connection reference"=w78) -> ("error out"=w84:errorcluster, "data"=w88:variant[][], "connection reference out"=w76:T16)  [unwired: 1 in]
      n7 = Variant To Data(error in=w84, type=string[][] [], Variant=w88) -> (data=w81:string[][], error out=w74:errorcluster)
      n8 = Index Array(array=w81) -> (element=w80:string[])  [unwired: 2 in]
      "SHIFT_DATA 2" <- w80
      n9 = Get Date/Time In Seconds() -> (seconds since 1Jan1904=w83:timestamp)
      n10 = call "String To Time_4.vi"("String Array In"=w80) -> ("Time Stamp Out"=w79:timestamp[])  [unwired: 9 in, 1 out]
      n11 = call "Shift Calculation_4.vi"("Current Time"=w83, "Time Stamp Out"=w79) -> ("Shift"=w75:i32)  [unwired: 8 in, 1 out]
    }
    frame True {
      n12 = call <vilib>:"DB Tools Select Data.vi"("condition"="where SNAME='D3'", "error in (no error)"=w96, "columns"=string[] ["AST", "AE", "BST", "BE", "CST", "CE"], "table"="SHIFT_TRAS", "connection reference"=w97) -> ("error out"=w101:errorcluster, "data"=w105:variant[][], "connection reference out"=w95:T16)  [unwired: 1 in]
      n13 = Variant To Data(error in=w101, type=string[][] [], Variant=w105) -> (data=w93:string[][], error out=w91:errorcluster)
      "appended array" <- w93
      n14 = Index Array(array=w93) -> (element=w92:string[])  [unwired: 2 in]
      "SHIFT_DATA" <- w92
      n15 = call "String To Time.vi"("error in (no error)"=w91, "String Array In"=w92) -> ("error out"=w90:errorcluster, "Time Stamp Out"=w98:timestamp[])  [unwired: 8 in]
      n16 = Get Date/Time In Seconds() -> (seconds since 1Jan1904=w100:timestamp)
      n17 = call "Shift Calculation.vi"("error in (no error)"=w90, "Current Time"=w100, "Time Stamp Out"=w98) -> ("error out"=w89:errorcluster, "Shift"=w99:i32)  [unwired: 7 in]
    }
  }
  n18 = control-ref of="This VI"() -> (w47:refnum<vi>)
  n19 = invoke class="VI" method="Default Vals.Reinit All"(reference=w47, error in=errorcluster {"status"=FALSE, "code"=0, "source"=""} ("error in (no error)")) -> (reference out=w46:refnum<vi>, error out=w4:errorcluster)  [unwired: 1 in, 1 out]
  n20 = case shown="3" w67 {
    tunnel: ["A" "B" "C" "D"] -> w60
    frame 1, Default {
    }
    frame 2 {
    }
    frame 3 {
    }
    frame 4 {
    }
  }
  n21 = local write "SHIFT"(w60) -> ()
  n22 = flat-sequence {
    tunnel: [w111] -> w5
    tunnel: w4 -> [w111]
    frame #0 {
      n23 = global write "DATA LOG.vi" "Auto Cycle On"(TRUE) -> ()
    }
  }
  n24 = global read "Global 1.vi" "BARCODE RECIPE"() -> (w13:string)
  n25 = call <vilib>:"DB Tools Select Data.vi"("error in (no error)"=w31, "columns"=string[] ["BARCODE_TRAC"], "table"="TRACEABILITY", "connection reference"=w32) -> ("error out"=w41:errorcluster, "data"=w40:variant[][], "connection reference out"=w19:T16)  [unwired: 2 in]
  n26 = call "PADMINI_varient_to_data.vi"("error in (no error)"=w41, "data"=w40) -> ("error out"=w17:errorcluster, "Array"=w39:string[][])  [unwired: 8 in]
  n27 = Index Array(array=w39, index (row)=0 ("disabled index (col)")) -> (element=w38:string[])  [unwired: 1 in]
  n28 = Format Into String(format string="where BARCODE_RECIPE='%s' ", w13) -> (resulting string=w11:string)  [unwired: 2 in, 1 out]
  n29 = Index Array(array=w38) -> (element=w34:string)  [unwired: 1 in]
  n30 = call <vilib>:"DB Tools Select Data.vi"("condition"=w11, "error in (no error)"=w17, "columns"=string[] ["BARCODE_RECIPE", "RECIPE_NAME"], "table"="BARCODE_RECIPE", "connection reference"=w19) -> ("error out"=w21:errorcluster, "data"=w20:variant[][], "connection reference out"=w18:T16)  [unwired: 1 in]
  n31 = To Upper Case(1:w34) -> (0:w33:string)
  n32 = Variant To Data(error in=w21, type=string[][] [], Variant=w20) -> (data=w14:string[][], error out=w16:errorcluster)
  n33 = case shown="\"False\", Default" w33 {
    tunnel: [FALSE ("BARCODE TRACEABILITY") TRUE ("BARCODE TRACEABILITY")] -> _
    tunnel: [0 1] -> w29
    frame "False", Default {
    }
    frame "TRUE" {
    }
  }
  n34 = Index Array(array=w14, index (col)=1 ("disabled index (col)")) -> (element=w9:string[])  [unwired: 1 in]
  n35 = Close Reference(reference=w46, error in (no error)=w5) -> (error out=w44:errorcluster)
  n36 = Index Array(array=w9) -> ()  [unwired: 1 in, 1 out]
  n37 = call "PADMINI_AUTO_TRACEABILITY_BYPASS.vi"("Enum"=enum16{"Read", "Write"}."Write", "error in (no error)"=w16, "I/P"=w29) -> ("error out"=w27:errorcluster)  [unwired: 7 in, 1 out]
  n38 = Obtain Queue(element data type=cluster{"CASE 2":T15} {"CASE 2"=enum."-1"}, error in (no error)=w44) -> (queue out=w71:refnum<queue>, error out=w24:errorcluster)  [unwired: 3 in, 1 out]
  n39 = flat-sequence {
    tunnel: w27 -> [w120]
    tunnel: [w120] -> w26
    frame #0 {
      w116 = FALSE
      n40 = global write "DATA LOG.vi" "ST 3 STRING 2"("" ("ST 3 STRING 2")) -> ()
      n41 = global write "DATA LOG.vi" "ST 4 STRING 3"("" ("ST 4 STRING 3")) -> ()
      n42 = global write "DATA LOG.vi" "OP30 ST 2 STRING"("" ("OP30 ST 2 STRING")) -> ()
      n43 = global write "DATA LOG.vi" "OP 100 reset"(w116) -> ()
      n44 = global write "DATA LOG.vi" "OP 110 reset"(w116) -> ()
      n45 = global write "DATA LOG.vi" "OP 30 reset"(w116) -> ()
      n46 = global write "DATA LOG.vi" "OP 50 reset"(w116) -> ()
      n47 = global write "DATA LOG.vi" "OP 70 reset"(w116) -> ()
      n48 = global write "DATA LOG.vi" "OP 80 reset"(w116) -> ()
      n49 = global write "DATA LOG.vi" "OP 90 reset"(w116) -> ()
      n50 = global write "DATA LOG.vi" "OP 20 reset"(w116) -> ()
      n51 = global write "DATA LOG.vi" "OP 40 reset"(w116) -> ()
      n52 = global write "DATA LOG.vi" "OP 60 reset"(w116) -> ()
      n53 = global write "DATA LOG.vi" "OP 20 Outputs"(w116) -> ()
      n54 = global write "DATA LOG.vi" "OP 10 Outputs"(w116) -> ()
      n55 = global write "DATA LOG.vi" "OP 30 Outputs"(w116) -> ()
      n56 = global write "DATA LOG.vi" "op 60"(0 ("op 30")) -> ()
      n57 = global write "DATA LOG.vi" "op 30"(0 ("op 30")) -> ()
      n58 = global write "DATA LOG.vi" "op 40"(0 ("op 30")) -> ()
    }
  }
  n59 = while {
    tunnel: w71 -> [w155]
    tunnel: w24 -> [w151]
    tunnel: w26 -> [w150]
    tunnel: w18 -> [w149]
    tunnel: [w125] -> w69
    tunnel: [w148] -> w2
    tunnel: FALSE -> [w147]
    tunnel: "REPORT" -> [w146]
    shift-right: [w144] -> _
    shift-left: string[] [] -> [w145]
    shift-right: [w143] -> _
    shift-left: "" ("trimmed string") -> [w142]
    shift-right: [w131] -> _
    shift-left: w3 -> [w140]
    stop <- w152 stop-if-true
    n60 = Dequeue Element(queue=w155, timeout in ms (-1)=250, error in (no error)=w151) -> (queue out=w128:refnum<queue>, element=w153:cluster{"CASE 2":T15}, error out=w154:errorcluster)  [unwired: 1 out]
    n61 = case shown="No Error" w154 {
      tunnel: w153 -> [w171 _]
      tunnel: [w167 TRUE] -> w152
      tunnel: w150 -> [w168 w1461]
      tunnel: w149 -> [w169 w1460]
      tunnel: [w165 w1461] -> w126
      tunnel: [w166 w1460] -> w148
      tunnel: w147 -> [w164 _]
      tunnel: w146 -> [w163 _]
      tunnel: w145 -> [w162 w1459]
      tunnel: [w161 w1459] -> w144
      tunnel: [w160 w1458] -> w143
      tunnel: w142 -> [w159 w1458]
      tunnel: w140 -> [w158 w1457]
      tunnel: [w157 w1457] -> w131
      tunnel: w128 -> [w156 _]
      frame No Error {
        n62 = Unbundle By Name(w171) -> ("CASE 2"=w170:T15)
        n63 = case shown="\"DATALOG1\"" w170 {
          tunnel: w169 -> [w242 w266 w334 w404 w457 w518 w572 w621 w670 w727 w776 w831 w880 w946 w992 w1039 w1088 w1136 w1185 w1234 w1274 w1354 w1435 w1444 w1452]
          tunnel: w168 -> [w239 w262 w311 w403 w444 w517 w558 w620 w656 w726 w763 w830 w866 w945 w981 w1038 w1075 w1135 w1171 w1233 w1273 w1336 w1421 w1443 w1454]
          tunnel: [FALSE FALSE FALSE FALSE FALSE FALSE FALSE FALSE FALSE FALSE FALSE FALSE FALSE FALSE FALSE FALSE FALSE FALSE FALSE FALSE FALSE FALSE FALSE FALSE TRUE] -> w167
          tunnel: [w242 w264 w331 w401 w454 w515 w569 w618 w667 w724 w773 w828 w877 w943 w989 w1036 w1086 w1133 w1182 w1231 w1271 w1351 w1433 w1444 w1451] -> w166
          tunnel: [w177 w244 w330 w398 w439 w512 w553 w615 w651 w721 w758 w825 w861 w940 w976 w1033 w1070 w1130 w1166 w1228 w1268 w1335 w1425 w1443 w1453] -> w165
          tunnel: w164 -> [_ w259 w333 w400 w456 w514 w571 w617 w669 w723 w775 w827 w879 w942 w991 w1035 w1069 w1132 w1184 w1230 w1270 w1353 _ _ _]
          tunnel: w163 -> [_ w265 w332 w402 w455 w516 w570 w619 w668 w725 w774 w829 w878 w944 w990 w1037 w1087 w1134 w1183 w1232 w1272 w1352 w1434 _ _]
          tunnel: w162 -> [w241 w263 w327 w395 w453 w510 w568 w613 w666 w719 w772 w823 w876 w938 w988 w1031 w1085 w1128 w1181 w1226 w1266 w1350 w1432 w1441 w1455]
          tunnel: [w241 w263 w327 w395 w453 w510 w568 w613 w666 w719 w772 w823 w876 w938 w988 w1031 w1085 w1128 w1181 w1226 w1266 w1350 w1432 w1441 w1455] -> w161
          tunnel: [w240 w258 w323 w396 w449 w509 w564 w612 w662 w718 w768 w822 w872 w937 w986 w1030 w1081 w1127 w1177 w1225 w1265 w1346 w1428 w1440 w1446] -> w160
          tunnel: w159 -> [w240 w258 w323 w396 w449 w509 w564 w612 w662 w718 w768 w822 w872 w937 w986 w1030 w1081 w1127 w1177 w1225 w1265 w1346 w1428 w1440 w1446]
          tunnel: w158 -> [w238 w252 w321 w394 w438 w508 w562 w611 w660 w717 w757 w821 w870 w936 w985 w1029 w1079 w1126 w1175 w1224 w1264 w1344 w1426 w1439 w1445]
          tunnel: [w181 w252 w321 w394 w438 w508 w562 w611 w660 w717 w757 w821 w870 w936 w985 w1029 w1079 w1126 w1175 w1224 w1264 w1344 w1426 w1439 w1445] -> w157
          tunnel: w156 -> [_ w246 _ _ _ _ _ _ _ _ _ _ _ _ _ _ _ _ _ _ _ _ _ _ _]
          frame "-1", Default {
            n64 = control-ref of="Final Result"() -> (w229:refnum<vi>)
            n65 = control-ref of="Top Result"() -> (w233:refnum<vi>)
            n66 = control-ref of="Bottom Result"() -> (w235:refnum<vi>)
            n67 = control-ref of="Camera Status"() -> (w234:refnum<vi>)
            n68 = control-ref of="Camera Status"() -> (w232:refnum<vi>)
            n69 = control-ref of="Final Result"() -> (w231:refnum<vi>)
            n70 = control-ref of="Final Result"() -> (w225:refnum<vi>)
            n71 = control-ref of="Shaft Status"() -> (w226:refnum<vi>)
            n72 = call "OP10 Indicators.vi"("error in (no error)"=w239, "OUTPUT INDICATOR"=w238, "Boolean in"=w229) -> ("error out"=w228:errorcluster, "OUTPUT INDICATOR"=w237:T13)  [unwired: 7 in]
            n73 = Build Array(w235, w234, w233, w232, w231) -> (w230:refnum<vi>[])
            n74 = Build Array(w226, w225) -> (w224:refnum<vi>[])
            n75 = control-ref of="RH Status"() -> (w221:refnum<vi>)
            n76 = control-ref of="Final Result"() -> (w175:refnum<vi>)
            n77 = control-ref of="LH Status"() -> (w220:refnum<vi>)
            n78 = control-ref of="Camera Status"() -> (w174:refnum<vi>)
            n79 = call "OP20 Indicators.vi"("error in (no error)"=w228, "Array"=w230, "OUTPUT INDICATOR"=w237) -> ("error out"=w227:errorcluster, "OUTPUT INDICATOR"=w236:T13)  [unwired: 7 in]
            n80 = control-ref of="Nut Status"() -> (w216:refnum<vi>)
            n81 = control-ref of="RH Status"() -> (w215:refnum<vi>)
            n82 = control-ref of="LH Status"() -> (w214:refnum<vi>)
            n83 = control-ref of="Camera Status"() -> (w213:refnum<vi>)
            n84 = control-ref of="Final Result"() -> (w212:refnum<vi>)
            n85 = Build Array(w221, w220, w174, w175) -> (w219:refnum<vi>[])
            n86 = call "OP30 Indicators.vi"("error in (no error)"=w227, "Array"=w224, "OUTPUT INDICATOR"=w236) -> ("error out"=w222:errorcluster, "OUTPUT INDICATOR"=w223:T13)  [unwired: 7 in]
            n87 = Build Array(w216, w215, w214, w213, w212) -> (w211:refnum<vi>[])
            n88 = call "OP40 Indicators.vi"("error in (no error)"=w222, "Array"=w219, "OUTPUT INDICATOR"=w223) -> ("error out"=w218:errorcluster, "OUTPUT INDICATOR"=w217:T13)  [unwired: 7 in]
            n89 = control-ref of="Screw 1 Status"() -> (w207:refnum<vi>)
            n90 = control-ref of="Screw 2 Status"() -> (w206:refnum<vi>)
            n91 = control-ref of="Screw 3 Status"() -> (w205:refnum<vi>)
            n92 = control-ref of="Screw 4 Status"() -> (w204:refnum<vi>)
            n93 = control-ref of="Screw 5 Status"() -> (w203:refnum<vi>)
            n94 = control-ref of="Screw 6 Status"() -> (w202:refnum<vi>)
            n95 = control-ref of="Final Result"() -> (w201:refnum<vi>)
            n96 = control-ref of="Final Result"() -> (w198:refnum<vi>)
            n97 = call "OP50 Indicators.vi"("error in (no error)"=w218, "Array"=w211, "OUTPUT INDICATOR"=w217) -> ("error out"=w210:errorcluster, "OUTPUT INDICATOR"=w209:T13)  [unwired: 7 in]
            n98 = Build Array(w207, w206, w205, w204, w203, w202, w201) -> (w208:refnum<vi>[])
            n99 = control-ref of="Loctite Status"() -> (w194:refnum<vi>)
            n100 = control-ref of="Final Result"() -> (w193:refnum<vi>)
            n101 = Build Array(w198) -> (w197:refnum<vi>[])
            n102 = call "OP60 Indicators.vi"("error in (no error)"=w210, "Array"=w208, "OUTPUT INDICATOR"=w209) -> ("error out"=w200:errorcluster, "OUTPUT INDICATOR"=w199:T13)  [unwired: 7 in]
            n103 = call "OP70 Indicators.vi"("error in (no error)"=w200, "Array"=w197, "OUTPUT INDICATOR"=w199) -> ("error out"=w196:errorcluster, "OUTPUT INDICATOR"=w195:T13)  [unwired: 7 in]
            n104 = control-ref of="Seat Status"() -> (w189:refnum<vi>)
            n105 = control-ref of="Final Result"() -> (w188:refnum<vi>)
            n106 = Build Array(w194, w193) -> (w192:refnum<vi>[])
            n107 = control-ref of="Final Result"() -> (w184:refnum<vi>)
            n108 = control-ref of="Camera Status"() -> (w176:refnum<vi>)
            n109 = call "OP80 Indicators.vi"("error in (no error)"=w196, "Array"=w192, "OUTPUT INDICATOR"=w195) -> ("error out"=w190:errorcluster, "OUTPUT INDICATOR"=w191:T13)  [unwired: 7 in]
            n110 = Build Array(w189, w188) -> (w187:refnum<vi>[])
            n111 = Build Array(w184, w176) -> (w183:refnum<vi>[])
            n112 = call "OP90 Indicators.vi"("error in (no error)"=w190, "Array"=w187, "OUTPUT INDICATOR"=w191) -> ("error out"=w186:errorcluster, "OUTPUT INDICATOR"=w185:T13)  [unwired: 7 in]
            n113 = call "OP100 Indicators.vi"("error in (no error)"=w186, "Array"=w183, "OUTPUT INDICATOR"=w185) -> ("error out"=w177:errorcluster, "OUTPUT INDICATOR"=w182:T13)  [unwired: 7 in]
            n114 = call "PADMINI_AUTO_BARCODE_STRING 110.vi"("Enum"=enum16{"Read", "Write"}."Read", "error in (no error)"=w177) -> ("Input 2"=w179:string[])  [unwired: 8 in, 1 out]
            n115 = Index Array(array=w179) -> (element #1=w180:string, element #2=w173:string, element #3=w172:string)  [unwired: 3 in]
            n116 = Bundle By Name(cluster=w182, "OP - 110.BARCODE"=w180, "OP - 110.BIN\nNumber"=w173, "OP - 110.PALLET\nNumber"=w172) -> (w181:T13)
          }
          frame "SCAN1" {
            # "STATION OP 10"
            n117 = global read "Global 1.vi" "BARCODE RECIPE"() -> (w253:string)
            n118 = call "PADMINI_AUTO_BARCODE_STRING.vi"("Enum"=enum16{"Read", "Write"}."Read", "error in (no error)"=w262) -> ("error out"=w261:errorcluster, "Input 2"=w249:string[])  [unwired: 8 in]
            n119 = Index Array(array=w249) -> (element=w248:string)  [unwired: 1 in]
            n120 = call <vilib>:"Trim Whitespace.vi"("string"=w248) -> ("trimmed string"=w247:string)  [unwired: 1 in]
            n121 = Match Pattern(string=w247, regular expression=w253) -> (match substring=w256:string)  [unwired: 1 in, 3 out]
            n122 = String Length(string=w253) -> (length=w255:i32)
            n123 = String Length(string=w256) -> (length=w254:i32)
            n124 = Equal?(x=w255, y=w254) -> (x = y?=w260:bool)
            n125 = case shown="False" w259 {
              tunnel: w266 -> [w292 w310]
              tunnel: w261 -> [w291 w308]
              tunnel: w265 -> [w290 _]
              tunnel: [w289 w307] -> w251
              tunnel: [w288 w310] -> w264
              tunnel: w260 -> [_ _]
              tunnel: w247 -> [w287 _]
              tunnel: [w286 TRUE] -> w245
              frame False {
                n126 = Format Into String(format string="where BARCODE='%s'", w287) -> (resulting string=w283:string)  [unwired: 2 in, 1 out]
                n127 = call <vilib>:"DB Tools Select Data.vi"("condition"=w283, "error in (no error)"=w291, "columns"=string[] ["BARCODE", "OP10_FINAL_RESULT"], "table"=w290, "connection reference"=w292) -> ("error out"=w282:errorcluster, "data"=w281:variant[][], "connection reference out"=w288:T16)  [unwired: 1 in]
                n128 = call "PADMINI_varient_to_data.vi"("error in (no error)"=w282, "data"=w281) -> ("error out"=w279:errorcluster, "Array"=w275:string[][])  [unwired: 8 in]
                n129 = Index Array(array=w275, index (row)=0) -> (element=→"SCAN OP10":string[])  [unwired: 1 in]
                n130 = Index Array(array=w275, index (row)=0, index (col)=1 ("index (row)")) -> (element=w276:string)
                n131 = Empty Array?(array=w275) -> (empty?=w280:bool)
                n132 = case shown="True" w280 {
                  tunnel: w279 -> [w302 w304]
                  tunnel: [w301 w304] -> w289
                  tunnel: [FALSE TRUE] -> w286
                  tunnel: w276 -> [w296 _]
                  frame False {
                    w295 = "OK"  # y
                    w298 = i32[] [1, 0]  # I/P
                    w297 = i32[] [0, 1]  # I/P
                    # "OP10 CURRENT STATION OK-NG\nPART REPEAT"
                    n133 = Equal?(x=w296, y=w295) -> (x = y?=w294:bool)
                    n134 = Select(t=w298, s=w294, f=w297) -> (s? t:f=w293:i32[])
                    "OP10 STATUS" <- w293
                    n135 = call "PADMINI_AUTO_BARCODE_STATUS.vi"("Enum"=enum16{"Read", "Write"}."Write", "error in (no error)"=w302, "I/P"=w293) -> ("error out"=w301:errorcluster)  [unwired: 7 in, 1 out]
                  }
                  frame True {
                    # "OP10 NEW part"
                  }
                }
              }
              frame True {
                w306 = i32[] [0, 1]  # I/P
                n136 = call "PADMINI_AUTO_BARCODE_STATUS.vi"("Enum"=enum16{"Read", "Write"}."Write", "error in (no error)"=w308, "I/P"=w306) -> ("error out"=w307:errorcluster)  [unwired: 7 in, 1 out]
              }
            }
            n137 = flat-sequence {
              tunnel: [w272] -> w250
              tunnel: w251 -> [w272]
              frame #0 {
                # "UPDATE op 10 sCAN sTATUS"
                n138 = global write "DATA LOG.vi" "OP 10 Outputs"(TRUE) -> ()
              }
            }
            n139 = call <vilib>:"Clear Errors.vi"("error in (no error)"=w250) -> ("error out"=w244:errorcluster)  [unwired: 5 in, 1 out]
            n140 = case shown="True" w245 {
              tunnel: w246 -> [_ w270]
              tunnel: w244 -> [_ w268]
              frame False {
              }
              frame True {
                w269 = cluster{"CASE 2":T15} {"CASE 2"=enum."DATALOG1"}  # element
                n141 = Enqueue Element(queue=w270, element=w269, error in (no error)=w268) -> ()  [unwired: 1 in, 3 out]
              }
            }
          }
          frame "DATALOG1" {
            w325 = T17 2 items=["no dialog", "OK message", "continue or stop message", "OK message + warnings", "continue/stop + warnings"] ("type of dialog (OK msg:1)")
            # "cycle result status\nwhether it was ok or nok\nor abortted in between"
            # "Printed QR Code data string"
            # "datalog of OP 10"
            n142 = call "PADMINI_AUTO_BARCODE_STRING.vi"("Enum"=enum16{"Read", "Write"}."Read", "error in (no error)"=w311) -> ("Input 2"=w318:string[])  [unwired: 8 in, 1 out]
            n143 = call "PADMINI_AUTO_CYCLE VALUE 10.vi"("Enum"=enum16{"Read", "Write"}."Read", "error in (no error)"=w311) -> ("error out"=w314:errorcluster, "Input 2"=w313:sgl[])  [unwired: 8 in]
            n144 = Index Array(array=w318) -> (element #1=w317:string, element #2=w316:string)  [unwired: 2 in]
            n145 = Index Array(array=w313) -> (element=w312:sgl)  [unwired: 1 in]
            n146 = Number To Fractional String(number=w312, precision (6)=i16 2) -> (F-format string=w319:string)  [unwired: 2 in]
            n147 = call <vilib>:"Trim Whitespace.vi"("string"=w317) -> ("trimmed string"=w328:string)  [unwired: 1 in]
            n148 = case shown="False" w333 {
              tunnel: w334 -> [w358 w393]
              tunnel: w314 -> [w360 w392]
              tunnel: [w366 w391] -> w331
              tunnel: [w365 w390] -> w326
              tunnel: w332 -> [w355 _]
              tunnel: w328 -> [w352 _]
              tunnel: w316 -> [w362 w383]
              tunnel: w319 -> [w346 w382]
              frame False {
                w354 = string[] ["BARCODE", "SHIFT", "OP10_DATE", "OP10_LEAK_RATE_SCCM", "OP10_FINAL_RESULT"]
                # "ST1 RESULT"
                # "DO TRACEBILITY"
                n149 = local read "SHIFT"() -> (w364:string)
                n150 = Format Into String(format string="Where BARCODE='%s' ", w352) -> (resulting string=w347:string)  [unwired: 2 in, 1 out]
                n151 = call <vilib>:"DB Tools Select Data.vi"("condition"=w347, "error in (no error)"=w360, "columns"=w354, "table"=w355, "connection reference"=w358) -> ("error out"=w356:errorcluster, "data"=w359:variant[][], "connection reference out"=w357:T16)  [unwired: 1 in]
                n152 = call "PADMINI_SHIFT_DATE.vi"("SHIFT"=w364) -> ("date/time string"=w363:string)  [unwired: 10 in]
                n153 = Variant To Data(error in=w356, type=string[][] [], Variant=w359) -> (data=w350:string[][], error out=w348:errorcluster)
                n154 = Bundle("trimmed string"=w352, "SHIFT"=w364, "date/time string"=w363, w346, "Input 2"=w362) -> (w361:T18)  [unwired: 1 in]
                n155 = Empty Array?(array=w350) -> (empty?=w349:bool)
                n156 = case shown="True" w349 {
                  tunnel: w357 -> [w371 w381]
                  tunnel: w348 -> [w370 w380]
                  tunnel: [w374 w379] -> w366
                  tunnel: [w373 w378] -> w365
                  tunnel: w354 -> [w368 w377]
                  tunnel: w355 -> [w369 w376]
                  tunnel: w361 -> [w372 w375]
                  tunnel: w347 -> [w367 _]
                  frame False {
                    n157 = call <vilib>:"DB Tools Update Data.vi"("condition"=w367, "data"=w372, "error in (no error)"=w370, "columns"=w368, "table"=w369, "connection reference"=w371) -> ("error out"=w373:errorcluster, "connection reference out"=w374:T16)  [unwired: 4 in]
                  }
                  frame True {
                    n158 = call <vilib>:"DB Tools Insert Data.vi"("data"=w375, "error in (no error)"=w380, "columns"=w377, "table"=w376, "connection reference"=w381) -> ("error out"=w378:errorcluster, "connection reference out"=w379:T16)  [unwired: 5 in]
                  }
                }
              }
              frame True {
                # "Trac BYPASS"
                n159 = local read "SHIFT"() -> (w388:string)
                n160 = call "PADMINI_SHIFT_DATE.vi"("SHIFT"=w388) -> ("date/time string"=w387:string)  [unwired: 10 in]
                n161 = Bundle("SHIFT"=w388, "date/time string"=w387, "Input 2"=w383, w382) -> (w386:T19)  [unwired: 1 in]
                n162 = To Variant(anything=w386) -> (Variant=w385:variant)
                n163 = call <vilib>:"DB Tools Insert Data.vi"("data"=w385, "error in (no error)"=w392, "columns"=string[] ["DATE", "SHIFT", "OP10_LEAK_RAT", "OP10_FINAL_RST"], "table"="ST1_REPORT", "connection reference"=w393) -> ("error out"=w390:errorcluster, "connection reference out"=w391:T16)  [unwired: 5 in]
              }
            }
            n164 = call <vilib>:"Simple Error Handler.vi"("type of dialog (OK msg:1)"=w325, "error in (no error)"=w326) -> ("error out"=w324:errorcluster)  [unwired: 3 in, 4 out]
            n165 = call <vilib>:"Clear Errors.vi"("error in (no error)"=w324) -> ("error out"=w322:errorcluster)  [unwired: 5 in, 1 out]
            n166 = disable-structure shown="Disabled" {
              disable-tunnel: [w344 w345] -> w330
              disable-tunnel: w322 -> [w343 w345]
              frame Disabled {
                w338 = refnum<vi> refnum  # Boolean
                n167 = property on="OP - 10" class="Clust"(error in=w343) -> (error out=w337:errorcluster, "Controls[]"=w341:refnum<vi>[])  [unwired: 1 in, 1 out]
                n168 = Index Array(array=w341, index=2) -> (element=w339:refnum<vi>)
                n169 = To More Specific Class(target class=w338, reference=w339, error in=w337) -> (specific class reference=w342:refnum<vi>, error out=w336:errorcluster)
                n170 = call "PADMINI_BOOL_COLOR_CHANGE.vi"("error in (no error)"=w336, "Boolean in"=w342) -> ("error out"=w344:errorcluster)  [unwired: 9 in]
              }
              frame Enabled {
              }
            }
          }
          frame "SCAN2" {
            # "Barcode Status\n0-Ideal, 1-Ok, 2-Nok, 3-Prev Station Not Done,\n4-Prev Station Nok,\n5- Already Done"
            # "STATION OP 20"
            n171 = case shown="False" w400 {
              tunnel: w404 -> [w429 w435]
              tunnel: w403 -> [w422 w433]
              tunnel: w402 -> [w410 _]
              tunnel: [w424 w432] -> w399
              tunnel: [w423 w435] -> w401
              tunnel: [w411 "" ("trimmed string")] -> _
              frame False {
                # "ST2 RESULT"
                # "ST1 RESULT"
                # "2 FOR EMPTY BARCODE READ OR MISMATCH"
                n172 = call "PADMINI_AUTO_BARCODE_STRING2.vi"("Enum"=enum16{"Read", "Write"}."Read", "error in (no error)"=w422) -> ("error out"=w421:errorcluster, "Input 2"=w413:string[])  [unwired: 8 in]
                n173 = global read "Global 1.vi" "BARCODE RECIPE"() -> (w414:string)
                n174 = Index Array(array=w413) -> (element=w412:string)  [unwired: 1 in]
                n175 = call <vilib>:"Trim Whitespace.vi"("string"=w412) -> ("trimmed string"=w411:string)  [unwired: 1 in]
                n176 = Match Pattern(string=w411, regular expression=w414) -> (match substring=w415:string)  [unwired: 1 in, 3 out]
                n177 = String Length(string=w414) -> (length=w417:i32)
                n178 = String Length(string=w415) -> (length=w416:i32)
                n179 = Format Into String(format string="WHERE BARCODE  ='%s'", w411) -> (resulting string=w418:string)  [unwired: 2 in, 1 out]
                n180 = Equal?(x=w417, y=w416) -> ()  [unwired: 1 out]
                n181 = call <vilib>:"DB Tools Select Data.vi"("condition"=w418, "error in (no error)"=w421, "columns"=string[] ["BARCODE", "OP10_FINAL_RESULT", "OP20_FINAL_RESULT"], "table"=w410, "connection reference"=w429) -> ("error out"=w427:errorcluster, "data"=w426:variant[][], "connection reference out"=w423:T16)  [unwired: 1 in]
                n182 = call "PADMINI_varient_to_data.vi"("error in (no error)"=w427, "data"=w426) -> ("error out"=w425:errorcluster, "Array"=w407:string[][])  [unwired: 8 in]
                n183 = Index Array(array=w407, index (row)=0 ("disabled index (col)")) -> (element=→"SCAN OP20":string[])  [unwired: 1 in]
                n184 = call "RESPONSE_LOGIC.vi"("Array"=w407) -> ("Not Found"=w405:i32[])  [unwired: 10 in]
                "OP20 STATUS" <- w405
                n185 = call "PADMINI_AUTO_BARCODE_STATUS 20.vi"("Enum"=enum16{"Read", "Write"}."Write", "error in (no error)"=w425, "I/P"=w405) -> ("error out"=w424:errorcluster)  [unwired: 7 in, 1 out]
              }
              frame True {
                w430 = i32[] [0, 0, 0, 0, 0]  # I/P
                n186 = call "PADMINI_AUTO_BARCODE_STATUS 20.vi"("Enum"=enum16{"Read", "Write"}."Write", "error in (no error)"=w433, "I/P"=w430) -> ("error out"=w432:errorcluster)  [unwired: 7 in, 1 out]
              }
            }
            n187 = flat-sequence {
              tunnel: [w437] -> w398
              tunnel: w399 -> [w437]
              frame #0 {
                # "UPDATE op 20 SCAN sTATUS"
                n188 = global write "DATA LOG.vi" "OP 20 Outputs"(TRUE) -> ()
              }
            }
          }
          frame "DATALOG2" {
            (unwired) string[] ["OP20_DATE", "OP20_LOWER_BEARING_DIS", "OP20_LOWER_BEARING_LOAD", "OP20_UPPER_BEARING_DIS", "OP20_UPPER_BEARING_LOAD", "OP20_LOWER_BEARING_RST", "OP20_BOTTOM_CAMERA_STATUS", "OP20_UPPER_SIM_STATUS", "OP20_UPPER_BERAING_RST", "OP20_UPPER_CAMERA_STATUS", "OP20_FINAL_RST"]
            w451 = T17 2 items=["no dialog", "OK message", "continue or stop message", "OK message + warnings", "continue/stop + warnings"] ("type of dialog (OK msg:1)")
            # "Printed QR Code data string"
            # "datalog of OP 20"
            n189 = call "PADMINI_AUTO_BARCODE_STRING2.vi"("Enum"=enum16{"Read", "Write"}."Read", "error in (no error)"=w444) -> ("error out"=w446:errorcluster, "Input 2"=w440:string[])  [unwired: 8 in]
            n190 = call "PADMINI_AUTO_CYCLE VALUE 20.vi"("Enum"=enum16{"Read", "Write"}."Read", "error in (no error)"=w444) -> ("Input 2"=w442:sgl[])  [unwired: 8 in, 1 out]
            n191 = Number To Fractional String(number=w442, precision (6)=i16 2) -> (F-format string=w441:string[])  [unwired: 2 in]
            n192 = case shown="False" w456 {
              tunnel: w457 -> [w481 w507]
              tunnel: w446 -> [w482 w506]
              tunnel: [w485 w505] -> w454
              tunnel: [w484 w504] -> w452
              tunnel: w455 -> [w480 _]
              tunnel: w441 -> [w477 w489]
              tunnel: w440 -> [w471 w490]
              frame False {
                # "ST2 RESULT"
                # "DO TRACEBILITY"
                n193 = Index Array(array=w471) -> (element #1=w472:string, element #2=w467:string, element #3=w466:string, element #4=w465:string, element #5=w464:string, element #6=w463:string, element #7=w462:string)  [unwired: 7 in]
                n194 = local read "SHIFT"() -> (w483:string)
                n195 = Index Array(array=w477) -> (element #1=w476:string, element #2=w475:string, element #3=w469:string, element #4=w468:string)  [unwired: 4 in]
                n196 = call <vilib>:"Trim Whitespace.vi"("string"=w472) -> ("trimmed string"=w473:string)  [unwired: 1 in]
                n197 = call "PADMINI_SHIFT_DATE.vi"("SHIFT"=w483) -> ("date/time string"=w470:string)  [unwired: 10 in]
                n198 = Format Into String(format string="Where BARCODE='%s' ", w473) -> (resulting string=w478:string)  [unwired: 2 in, 1 out]
                n199 = Bundle("date/time string"=w470, "Input 2"=w476, "Input 2"=w475, "Input 2"=w469, "Input 2"=w468, "Input 2"=w467, "Input 2"=w466, "Input 2"=w465, "Input 2"=w464, "Input 2"=w463, "Input 2"=w462) -> (w474:T20)  [unwired: 1 in]
                n200 = call <vilib>:"DB Tools Update Data.vi"("condition"=w478, "data"=w474, "error in (no error)"=w482, "columns"=string[] ["OP20_DATE", "OP20_BOTTOM_DISPLACE_mm", "OP20_BOTTOM_LOAD_kg", "OP20_TOP_DISPLACE_mm", "OP20_TOP_LOAD_kg", "OP20_BOTTOM_RESULT", "OP20_BOTTOM_CAMERA_STATUS", "OP20_TOP_SIM_STATUS", "OP20_TOP_RESULT", "OP20_TOP_CAMERA_STATUS", "OP20_FINAL_RESULT"], "table"=w480, "connection reference"=w481) -> ("error out"=w484:errorcluster, "connection reference out"=w485:T16)  [unwired: 4 in]
              }
              frame True {
                n201 = local read "SHIFT"() -> (w487:string)
                n202 = Index Array(array=w490) -> (element #2=w496:string, element #3=w495:string, element #4=w494:string, element #5=w493:string, element #6=w492:string, element #7=w486:string)  [unwired: 7 in, 1 out]
                n203 = call "PADMINI_SHIFT_DATE.vi"("SHIFT"=w487) -> ("date/time string"=w488:string)  [unwired: 10 in]
                n204 = Index Array(array=w489) -> (element #1=w500:string, element #2=w499:string, element #3=w498:string, element #4=w497:string)  [unwired: 4 in]
                n205 = Bundle("date/time string"=w488, "SHIFT"=w487, "Input 2"=w500, "Input 2"=w499, "Input 2"=w496, "Input 2"=w495, "Input 2"=w498, "Input 2"=w497, "Input 2"=w494, "Input 2"=w493, "Input 2"=w492, "Input 2"=w486) -> (w491:T21)  [unwired: 1 in]
                n206 = To Variant(anything=w491) -> (Variant=w502:variant)
                n207 = call <vilib>:"DB Tools Insert Data.vi"("data"=w502, "error in (no error)"=w506, "columns"=string[] ["DATE", "SHIFT", "ST2_LOWER_BEARING_DIS", "ST2_LOWER_BEARING_LOAD", "ST2_BOTTOM_CAMERA_STATUS", "ST2_LOWER_BEARING_RST", "ST2_UPPER_BEARING_DIS", "ST2_UPPER_BEARING_LOAD", "ST2_UPPER_SIM_STATUS", "ST2_UPPER_CAMERA_STATUS", "ST2_UPPER_BERAING_RST", "ST2_FINAL_RST"], "table"="ST2_REPORT", "connection reference"=w507) -> ("error out"=w504:errorcluster, "connection reference out"=w505:T16)  [unwired: 5 in]
              }
            }
            n208 = call <vilib>:"Simple Error Handler.vi"("type of dialog (OK msg:1)"=w451, "error in (no error)"=w452) -> ("error out"=w450:errorcluster)  [unwired: 3 in, 4 out]
            n209 = call <vilib>:"Clear Errors.vi"("error in (no error)"=w450) -> ("error out"=w448:errorcluster)  [unwired: 5 in, 1 out]
            n210 = flat-sequence {
              tunnel: [w460] -> w439
              tunnel: w448 -> [w460]
              frame #0 {
                # "UPDATE op 20 save"
                n211 = global write "DATA LOG.vi" "OP 20 reset"(TRUE) -> ()
              }
            }
          }
          frame "SCAN3" {
            # "STATION OP 30"
            n212 = case shown="False" w514 {
              tunnel: w518 -> [w544 w550]
              tunnel: w517 -> [w537 w548]
              tunnel: w516 -> [w524 _]
              tunnel: [w539 w547] -> w513
              tunnel: [w538 w550] -> w515
              tunnel: [w525 "" ("trimmed string")] -> _
              frame False {
                n213 = call "PADMINI_AUTO_BARCODE_STRING 30.vi"("Enum"=enum16{"Read", "Write"}."Read", "error in (no error)"=w537) -> ("error out"=w536:errorcluster, "Input 2"=w527:string[])  [unwired: 8 in]
                n214 = global read "Global 1.vi" "BARCODE RECIPE"() -> (w528:string)
                n215 = Index Array(array=w527) -> (element=w526:string)  [unwired: 1 in]
                n216 = call <vilib>:"Trim Whitespace.vi"("string"=w526) -> ("trimmed string"=w525:string)  [unwired: 1 in]
                n217 = Match Pattern(string=w525, regular expression=w528) -> (match substring=w529:string)  [unwired: 1 in, 3 out]
                n218 = String Length(string=w528) -> (length=w531:i32)
                n219 = String Length(string=w529) -> (length=w530:i32)
                n220 = Equal?(x=w525, y="") -> ()  [unwired: 1 out]
                n221 = Format Into String(format string="WHERE BARCODE  ='%s'", w525) -> (resulting string=w533:string)  [unwired: 2 in, 1 out]
                n222 = Equal?(x=w531, y=w530) -> ()  [unwired: 1 out]
                n223 = call <vilib>:"DB Tools Select Data.vi"("condition"=w533, "error in (no error)"=w536, "columns"=string[] ["BARCODE", "OP20_FINAL_RESULT", "OP30_FINAL_RESULT"], "table"=w524, "connection reference"=w544) -> ("error out"=w542:errorcluster, "data"=w541:variant[][], "connection reference out"=w538:T16)  [unwired: 1 in]
                n224 = call "PADMINI_varient_to_data.vi"("error in (no error)"=w542, "data"=w541) -> ("error out"=w540:errorcluster, "Array"=w521:string[][])  [unwired: 8 in]
                n225 = Index Array(array=w521, index (row)=0 ("disabled index (col)")) -> (element=→"SCAN OP30":string[])  [unwired: 1 in]
                n226 = call "RESPONSE_LOGIC.vi"("Array"=w521) -> ("Not Found"=w519:i32[])  [unwired: 10 in]
                "OP30 STATUS" <- w519
                n227 = call "PADMINI_AUTO_BARCODE_STATUS 30.vi"("Enum"=enum16{"Read", "Write"}."Write", "error in (no error)"=w540, "I/P"=w519) -> ("error out"=w539:errorcluster)  [unwired: 7 in, 1 out]
              }
              frame True {
                w545 = i32[] [0, 0, 0, 0, 0]  # I/P
                n228 = call "PADMINI_AUTO_BARCODE_STATUS 30.vi"("Enum"=enum16{"Read", "Write"}."Write", "error in (no error)"=w548, "I/P"=w545) -> ("error out"=w547:errorcluster)  [unwired: 7 in, 1 out]
              }
            }
            n229 = flat-sequence {
              tunnel: [w552] -> w512
              tunnel: w513 -> [w552]
              frame #0 {
                # "UPDATE op 30 SCAN sTATUS"
                n230 = global write "DATA LOG.vi" "OP 30 Outputs"(TRUE) -> ()
              }
            }
          }
          frame "DATALOG3" {
            (unwired) string[] ["OP30_DATE", "OP30_DISPLACEMENT", "OP30_SHAFT_PRESS_LOAD", "OP30_SHAFT_STATUS", "OP30_FINAL_RST"]
            w566 = T17 2 items=["no dialog", "OK message", "continue or stop message", "OK message + warnings", "continue/stop + warnings"] ("type of dialog (OK msg:1)")
            # "Printed QR Code data string"
            # "datalog of OP 30"
            n231 = call "PADMINI_AUTO_BARCODE_STRING 30.vi"("Enum"=enum16{"Read", "Write"}."Read", "error in (no error)"=w558) -> ("error out"=w560:errorcluster, "Input 2"=w554:string[])  [unwired: 8 in]
            n232 = call "PADMINI_AUTO_CYCLE VALUE 30.vi"("Enum"=enum16{"Read", "Write"}."Read", "error in (no error)"=w558) -> ("Input 2"=w556:sgl[])  [unwired: 8 in, 1 out]
            n233 = Number To Fractional String(number=w556, precision (6)=i16 2) -> (F-format string=w555:string[])  [unwired: 2 in]
            n234 = case shown="False" w571 {
              tunnel: w572 -> [w590 w610]
              tunnel: w560 -> [w591 w609]
              tunnel: [w594 w608] -> w569
              tunnel: [w593 w607] -> w567
              tunnel: w570 -> [w589 _]
              tunnel: w555 -> [w586 w595]
              tunnel: w554 -> [w580 w596]
              frame False {
                # "DO TRACEBILITY"
                n235 = Index Array(array=w580) -> (element #1=w581:string, element #2=w579:string, element #3=w578:string)  [unwired: 3 in]
                n236 = local read "SHIFT"() -> (w592:string)
                n237 = Index Array(array=w586) -> (element #1=w585:string, element #2=w584:string)  [unwired: 2 in]
                n238 = call <vilib>:"Trim Whitespace.vi"("string"=w581) -> ("trimmed string"=w582:string)  [unwired: 1 in]
                n239 = call "PADMINI_SHIFT_DATE.vi"("SHIFT"=w592) -> ("date/time string"=w577:string)  [unwired: 10 in]
                n240 = Format Into String(format string="Where BARCODE='%s' ", w582) -> (resulting string=w587:string)  [unwired: 2 in, 1 out]
                n241 = Bundle("date/time string"=w577, "Input 2"=w585, "Input 2"=w584, "Input 2"=w579, "Input 2"=w578) -> (w583:T22)  [unwired: 1 in]
                n242 = call <vilib>:"DB Tools Update Data.vi"("condition"=w587, "data"=w583, "error in (no error)"=w591, "columns"=string[] ["OP30_DATE", "OP30_DISPLACEMENT_mm", "OP30_SHAFT_PRESS_LOAD_kg", "OP30_SHAFT_STATUS", "OP30_FINAL_RESULT"], "table"=w589, "connection reference"=w590) -> ("error out"=w593:errorcluster, "connection reference out"=w594:T16)  [unwired: 4 in]
              }
              frame True {
                # "TRAC BYPASS"
                n243 = local read "SHIFT"() -> (w597:string)
                n244 = call "PADMINI_SHIFT_DATE.vi"("SHIFT"=w597) -> ("date/time string"=w598:string)  [unwired: 10 in]
                n245 = Index Array(array=w596) -> (element #2=w602:string, element #3=w601:string)  [unwired: 3 in, 1 out]
                n246 = Index Array(array=w595) -> (element #1=w604:string, element #2=w603:string)  [unwired: 2 in]
                n247 = Bundle("date/time string"=w598, "SHIFT"=w597, "Input 2"=w604, "Input 2"=w603, "Input 2"=w602, "Input 2"=w601) -> (w599:T23)  [unwired: 1 in]
                n248 = To Variant(anything=w599) -> (Variant=w600:variant)
                n249 = call <vilib>:"DB Tools Insert Data.vi"("data"=w600, "error in (no error)"=w609, "columns"=string[] ["DATE", "SHIFT", "ST3_DISPLACEMENT", "ST3_LOAD", "ST3_MIDDLE_GEAR_SHAFT_STATUS", "ST3_FINAL_RST"], "table"="ST3_REPORT", "connection reference"=w610) -> ("error out"=w607:errorcluster, "connection reference out"=w608:T16)  [unwired: 5 in]
              }
            }
            n250 = call <vilib>:"Simple Error Handler.vi"("type of dialog (OK msg:1)"=w566, "error in (no error)"=w567) -> ("error out"=w565:errorcluster)  [unwired: 3 in, 4 out]
            n251 = call <vilib>:"Clear Errors.vi"("error in (no error)"=w565) -> ("error out"=w563:errorcluster)  [unwired: 5 in, 1 out]
            n252 = flat-sequence {
              tunnel: [w575] -> w553
              tunnel: w563 -> [w575]
              frame #0 {
                # "UPDATE op 20 save"
                n253 = global write "DATA LOG.vi" "OP 30 reset"(TRUE) -> ()
              }
            }
          }
          frame "SCAN4" {
            # "STATION OP 40"
            n254 = case shown="False" w617 {
              tunnel: w621 -> [w642 w648]
              tunnel: w620 -> [w635 w647]
              tunnel: w619 -> [w627 _]
              tunnel: [w637 w646] -> w616
              tunnel: [w636 w648] -> w618
              tunnel: [w628 "" ("trimmed string")] -> _
              frame False {
                n255 = call "PADMINI_AUTO_BARCODE_STRING 40.vi"("Enum"=enum16{"Read", "Write"}."Read", "error in (no error)"=w635) -> ("error out"=w634:errorcluster, "Input 2"=w630:string[])  [unwired: 8 in]
                n256 = Index Array(array=w630) -> (element=w629:string)  [unwired: 1 in]
                n257 = call <vilib>:"Trim Whitespace.vi"("string"=w629) -> ("trimmed string"=w628:string)  [unwired: 1 in]
                n258 = Format Into String(format string="WHERE BARCODE  ='%s'", w628) -> (resulting string=w631:string)  [unwired: 2 in, 1 out]
                n259 = call <vilib>:"DB Tools Select Data.vi"("condition"=w631, "error in (no error)"=w634, "columns"=string[] ["BARCODE", "OP30_FINAL_RESULT", "OP40_FINAL_RESULT"], "table"=w627, "connection reference"=w642) -> ("error out"=w640:errorcluster, "data"=w639:variant[][], "connection reference out"=w636:T16)  [unwired: 1 in]
                n260 = call "PADMINI_varient_to_data.vi"("error in (no error)"=w640, "data"=w639) -> ("error out"=w638:errorcluster, "Array"=w624:string[][])  [unwired: 8 in]
                n261 = call "RESPONSE_LOGIC.vi"("Array"=w624) -> ("Not Found"=w622:i32[])  [unwired: 10 in]
                "OP40 STATUS" <- w622
                n262 = Index Array(array=w624, index (row)=0 ("disabled index (col)")) -> (element=→"SCAN OP40":string[])  [unwired: 1 in]
                n263 = call "PADMINI_AUTO_BARCODE_STATUS 40.vi"("Enum"=enum16{"Read", "Write"}."Write", "error in (no error)"=w638, "I/P"=w622) -> ("error out"=w637:errorcluster)  [unwired: 7 in, 1 out]
              }
              frame True {
                w643 = i32[] [0, 0, 0, 0, 0]  # I/P
                n264 = call "PADMINI_AUTO_BARCODE_STATUS 40.vi"("Enum"=enum16{"Read", "Write"}."Write", "error in (no error)"=w647, "I/P"=w643) -> ("error out"=w646:errorcluster)  [unwired: 7 in, 1 out]
              }
            }
            n265 = flat-sequence {
              tunnel: [w650] -> w615
              tunnel: w616 -> [w650]
              frame #0 {
                # "UPDATE op 40 SCAN sTATUS"
                n266 = global write "DATA LOG.vi" "OP 40 Outputs"(TRUE) -> ()
              }
            }
          }
          frame "DATALOG4" {
            w664 = T17 2 items=["no dialog", "OK message", "continue or stop message", "OK message + warnings", "continue/stop + warnings"] ("type of dialog (OK msg:1)")
            # "datalog of OP 40"
            n267 = call "PADMINI_AUTO_BARCODE_STRING 40.vi"("Enum"=enum16{"Read", "Write"}."Read", "error in (no error)"=w656) -> ("error out"=w658:errorcluster, "Input 2"=w652:string[])  [unwired: 8 in]
            n268 = call "PADMINI_AUTO_CYCLE VALUE 40.vi"("Enum"=enum16{"Read", "Write"}."Read", "error in (no error)"=w656) -> ("Input 2"=w654:sgl[])  [unwired: 8 in, 1 out]
            n269 = Number To Fractional String(number=w654, precision (6)=i16 2) -> (F-format string=w653:string[])  [unwired: 2 in]
            n270 = case shown="False" w669 {
              tunnel: w670 -> [w692 w716]
              tunnel: w658 -> [w693 w715]
              tunnel: [w696 w714] -> w667
              tunnel: [w695 w713] -> w665
              tunnel: w668 -> [w691 _]
              tunnel: w653 -> [w687 w698]
              tunnel: w652 -> [w682 w697]
              frame False {
                # "DO TRACEBILITY"
                n271 = Index Array(array=w682) -> (element #1=w683:string, element #2=w678:string, element #3=w677:string, element #4=w675:string, element #5=w674:string)  [unwired: 5 in]
                n272 = local read "SHIFT"() -> (w694:string)
                n273 = Index Array(array=w687) -> (element #1=w686:string, element #2=w681:string, element #3=w680:string, element #4=w679:string)  [unwired: 4 in]
                n274 = call <vilib>:"Trim Whitespace.vi"("string"=w683) -> ("trimmed string"=w684:string)  [unwired: 1 in]
                n275 = call "PADMINI_SHIFT_DATE.vi"("SHIFT"=w694) -> ("date/time string"=w676:string)  [unwired: 10 in]
                n276 = Format Into String(format string="Where BARCODE='%s' ", w684) -> (resulting string=w689:string)  [unwired: 2 in, 1 out]
                n277 = Bundle("date/time string"=w676, "Input 2"=w686, "Input 2"=w678, "Input 2"=w681, "Input 2"=w677, "Input 2"=w680, "Input 2"=w679, "Input 2"=w675, "Input 2"=w674) -> (w685:T24)  [unwired: 1 in]
                n278 = call <vilib>:"DB Tools Update Data.vi"("condition"=w689, "data"=w685, "error in (no error)"=w693, "columns"=string[] ["OP40_DATE", "OP40_RH_SCREW_Nm", "OP40_RH_STATUS", "OP40_LH_SCREW_Nm", "OP40_LH_STATUS", "OP40_DISPLACEMENT_mm", "OP40_STACK_LOAD_kg", "OP40_TOP_BEARING_CAMERA_STAUS", "OP40_FINAL_RESULT"], "table"=w691, "connection reference"=w692) -> ("error out"=w695:errorcluster, "connection reference out"=w696:T16)  [unwired: 4 in]
              }
              frame True {
                # "TRAC BYPASS"
                n279 = local read "SHIFT"() -> (w699:string)
                n280 = Index Array(array=w697) -> (element #2=w707:string, element #3=w706:string, element #4=w705:string, element #5=w704:string)  [unwired: 5 in, 1 out]
                n281 = call "PADMINI_SHIFT_DATE.vi"("SHIFT"=w699) -> ("date/time string"=w700:string)  [unwired: 10 in]
                n282 = Index Array(array=w698) -> (element #1=w701:string, element #2=w710:string, element #3=w709:string, element #4=w708:string)  [unwired: 4 in]
                n283 = Bundle("date/time string"=w700, "SHIFT"=w699, "Input 2"=w701, "Input 2"=w707, "Input 2"=w710, "Input 2"=w706, "Input 2"=w709, "Input 2"=w708, "Input 2"=w704, "Input 2"=w705) -> (w703:T25)  [unwired: 1 in]
                n284 = To Variant(anything=w703) -> (Variant=w702:variant)
                n285 = call <vilib>:"DB Tools Insert Data.vi"("data"=w702, "error in (no error)"=w715, "columns"=string[] ["DATE", "SHIFT", "ST4_SCREW1_DATA", "ST4_SCREW1_STATUS", "ST4_SCREW2_DATA", "ST4_SCREW2_STATUS", "ST4_DISPLACEMENT", "ST4_LOAD", "ST4_TOP_BEARING_CAMERA_STAUS", "ST4_FINAL_RST"], "table"="ST4_REPORT", "connection reference"=w716) -> ("error out"=w713:errorcluster, "connection reference out"=w714:T16)  [unwired: 5 in]
              }
            }
            n286 = call <vilib>:"Simple Error Handler.vi"("type of dialog (OK msg:1)"=w664, "error in (no error)"=w665) -> ("error out"=w663:errorcluster)  [unwired: 3 in, 4 out]
            n287 = call <vilib>:"Clear Errors.vi"("error in (no error)"=w663) -> ("error out"=w661:errorcluster)  [unwired: 5 in, 1 out]
            n288 = flat-sequence {
              tunnel: [w673] -> w651
              tunnel: w661 -> [w673]
              frame #0 {
                # "UPDATE op 20 save"
                n289 = global write "DATA LOG.vi" "OP 40 reset"(TRUE) -> ()
              }
            }
          }
          frame "SCAN5" {
            # "STATION OP 50"
            n290 = case shown="False" w723 {
              tunnel: w727 -> [w748 w754]
              tunnel: w726 -> [w741 w753]
              tunnel: w725 -> [w733 _]
              tunnel: [w743 w752] -> w722
              tunnel: [w742 w754] -> w724
              tunnel: [w734 "" ("trimmed string")] -> _
              frame False {
                n291 = call "PADMINI_AUTO_BARCODE_STRING 50.vi"("Enum"=enum16{"Read", "Write"}."Read", "error in (no error)"=w741) -> ("error out"=w740:errorcluster, "Input 2"=w736:string[])  [unwired: 8 in]
                n292 = Index Array(array=w736) -> (element=w735:string)  [unwired: 1 in]
                n293 = call <vilib>:"Trim Whitespace.vi"("string"=w735) -> ("trimmed string"=w734:string)  [unwired: 1 in]
                n294 = Format Into String(format string="WHERE BARCODE  ='%s'", w734) -> (resulting string=w737:string)  [unwired: 2 in, 1 out]
                n295 = call <vilib>:"DB Tools Select Data.vi"("condition"=w737, "error in (no error)"=w740, "columns"=string[] ["BARCODE", "OP40_FINAL_RESULT", "OP50_FINAL_RESULT"], "table"=w733, "connection reference"=w748) -> ("error out"=w746:errorcluster, "data"=w745:variant[][], "connection reference out"=w742:T16)  [unwired: 1 in]
                n296 = call "PADMINI_varient_to_data.vi"("error in (no error)"=w746, "data"=w745) -> ("error out"=w744:errorcluster, "Array"=w730:string[][])  [unwired: 8 in]
                n297 = Index Array(array=w730, index (row)=0 ("disabled index (col)")) -> (element=→"SCAN OP50":string[])  [unwired: 1 in]
                n298 = call "RESPONSE_LOGIC.vi"("Array"=w730) -> ("Not Found"=w729:i32[])  [unwired: 10 in]
                "OP50 STATUS" <- w729
                n299 = call "PADMINI_AUTO_BARCODE_STATUS 50.vi"("Enum"=enum16{"Read", "Write"}."Write", "error in (no error)"=w744, "I/P"=w729) -> ("error out"=w743:errorcluster)  [unwired: 7 in, 1 out]
              }
              frame True {
                w749 = i32[] [0, 0, 0, 0, 0]  # I/P
                n300 = call "PADMINI_AUTO_BARCODE_STATUS 50.vi"("Enum"=enum16{"Read", "Write"}."Write", "error in (no error)"=w753, "I/P"=w749) -> ("error out"=w752:errorcluster)  [unwired: 7 in, 1 out]
              }
            }
            n301 = flat-sequence {
              tunnel: [w756] -> w721
              tunnel: w722 -> [w756]
              frame #0 {
                # "UPDATE op 50 SCAN sTATUS"
                n302 = global write "DATA LOG.vi" "OP 50 Outputs"(TRUE) -> ()
              }
            }
          }
          frame "DATALOG5" {
            (unwired) string[] ["OP50_DATE", "OP50_NUT_TORQUE_Nm", "OP50_NUT_STATUS", "OP50_LH_MOTOR_SCREW_Nm", "OP50_LH_STATUS", "OP50_RH_MOTOR_SCREW_Nm", "OP50_RH_STATUS", "OP50_CAMERA_STATUS", "OP50_FINAL_RESULT"]
            w770 = T17 2 items=["no dialog", "OK message", "continue or stop message", "OK message + warnings", "continue/stop + warnings"] ("type of dialog (OK msg:1)")
            # "datalog of OP 50"
            n303 = call "PADMINI_AUTO_BARCODE_STRING 50.vi"("Enum"=enum16{"Read", "Write"}."Read", "error in (no error)"=w763) -> ("error out"=w765:errorcluster, "Input 2"=w759:string[])  [unwired: 8 in]
            n304 = call "PADMINI_AUTO_CYCLE VALUE 50.vi"("Enum"=enum16{"Read", "Write"}."Read", "error in (no error)"=w763) -> ("Input 2"=w761:sgl[])  [unwired: 8 in, 1 out]
            n305 = Number To Fractional String(number=w761, precision (6)=i16 2) -> (F-format string=w760:string[])  [unwired: 2 in]
            n306 = case shown="False" w775 {
              tunnel: w776 -> [w798 w820]
              tunnel: w765 -> [w799 w819]
              tunnel: [w802 w818] -> w773
              tunnel: [w801 w817] -> w771
              tunnel: w774 -> [w797 _]
              tunnel: w760 -> [w794 w804]
              tunnel: w759 -> [w790 w803]
              frame False {
                # "DO TRACEBILITY"
                n307 = Index Array(array=w790) -> (element #1=w791:string, element #2=w786:string, element #3=w784:string, element #4=w782:string, element #5=w781:string, element #6=w780:string)  [unwired: 6 in]
                n308 = local read "SHIFT"() -> (w800:string)
                n309 = Index Array(array=w794) -> (element #1=w787:string, element #2=w785:string, element #3=w783:string)  [unwired: 3 in]
                n310 = call <vilib>:"Trim Whitespace.vi"("string"=w791) -> ("trimmed string"=w792:string)  [unwired: 1 in]
                n311 = call "PADMINI_SHIFT_DATE.vi"("SHIFT"=w800) -> ("date/time string"=w789:string)  [unwired: 10 in]
                n312 = Format Into String(format string="Where BARCODE='%s' ", w792) -> (resulting string=w795:string)  [unwired: 2 in, 1 out]
                n313 = Bundle("date/time string"=w789, "Input 2"=w787, "Input 2"=w786, "Input 2"=w785, "Input 2"=w784, "Input 2"=w783, "Input 2"=w782, "Input 2"=w781, "Input 2"=w780) -> (w793:T24)  [unwired: 1 in]
                n314 = call <vilib>:"DB Tools Update Data.vi"("condition"=w795, "data"=w793, "error in (no error)"=w799, "columns"=string[] ["OP50_DATE", "OP50_NUT_TORQUE_Nm", "OP50_NUT_STATUS", "OP50_RH_MOTOR_SCREW_Nm", "OP50_RH_STATUS", "OP50_LH_MOTOR_SCREW_Nm", "OP50_LH_STATUS", "OP50_CAMERA_STATUS", "OP50_FINAL_RESULT"], "table"=w797, "connection reference"=w798) -> ("error out"=w801:errorcluster, "connection reference out"=w802:T16)  [unwired: 4 in]
              }
              frame True {
                # "TRAC BYPASS"
                n315 = local read "SHIFT"() -> (w805:string)
                n316 = Index Array(array=w803) -> (element #2=w809:string, element #3=w808:string, element #4=w813:string)  [unwired: 4 in, 1 out]
                n317 = Index Array(array=w804) -> (element #1=w812:string, element #2=w811:string, element #3=w810:string)  [unwired: 3 in]
                n318 = call "PADMINI_SHIFT_DATE.vi"("SHIFT"=w805) -> ("date/time string"=w806:string)  [unwired: 10 in]
                n319 = Bundle("date/time string"=w806, "SHIFT"=w805, "Input 2"=w812, "Input 2"=w809, "Input 2"=w811, "Input 2"=w808, "Input 2"=w810, "Input 2"=w813) -> (w807:T26)  [unwired: 1 in]
                n320 = To Variant(anything=w807) -> (Variant=w816:variant)
                n321 = call <vilib>:"DB Tools Insert Data.vi"("data"=w816, "error in (no error)"=w819, "columns"=string[] ["DATE", "SHIFT", "ST5_SCREW1_DATA", "ST5_SCREW1_STATUS", "ST5_SCREW2_DATA", "ST5_SCREW2_STATUS", "ST5_SCREW3_DATA", "ST5_FINAL_RST"], "table"="ST5_REPORT", "connection reference"=w820) -> ("error out"=w817:errorcluster, "connection reference out"=w818:T16)  [unwired: 5 in]
              }
            }
            n322 = call <vilib>:"Simple Error Handler.vi"("type of dialog (OK msg:1)"=w770, "error in (no error)"=w771) -> ("error out"=w769:errorcluster)  [unwired: 3 in, 4 out]
            n323 = call <vilib>:"Clear Errors.vi"("error in (no error)"=w769) -> ("error out"=w767:errorcluster)  [unwired: 5 in, 1 out]
            n324 = flat-sequence {
              tunnel: [w779] -> w758
              tunnel: w767 -> [w779]
              frame #0 {
                # "UPDATE op 20 save"
                n325 = global write "DATA LOG.vi" "OP 50 reset"(TRUE) -> ()
              }
            }
          }
          frame "SCAN6" {
            # "STATION OP 60"
            n326 = case shown="False" w827 {
              tunnel: w831 -> [w852 w858]
              tunnel: w830 -> [w845 w857]
              tunnel: w829 -> [_ _]
              tunnel: [w847 w856] -> w826
              tunnel: [w846 w858] -> w828
              tunnel: [w837 "" ("trimmed string")] -> _
              frame False {
                n327 = call "PADMINI_AUTO_BARCODE_STRING 60.vi"("Enum"=enum16{"Read", "Write"}."Read", "error in (no error)"=w845) -> ("error out"=w844:errorcluster, "Input 2"=w839:string[])  [unwired: 8 in]
                n328 = Index Array(array=w839) -> (element=w838:string)  [unwired: 1 in]
                n329 = call <vilib>:"Trim Whitespace.vi"("string"=w838) -> ("trimmed string"=w837:string)  [unwired: 1 in]
                n330 = Format Into String(format string="WHERE BARCODE  ='%s'", w837) -> (resulting string=w840:string)  [unwired: 2 in, 1 out]
                n331 = call <vilib>:"DB Tools Select Data.vi"("condition"=w840, "error in (no error)"=w844, "columns"=string[] ["BARCODE", "OP50_FINAL_RESULT", "OP60_FINAL_RESULT"], "table"="REPORT", "connection reference"=w852) -> ("error out"=w850:errorcluster, "data"=w849:variant[][], "connection reference out"=w846:T16)  [unwired: 1 in]
                n332 = call "PADMINI_varient_to_data.vi"("error in (no error)"=w850, "data"=w849) -> ("error out"=w848:errorcluster, "Array"=w834:string[][])  [unwired: 8 in]
                n333 = Index Array(array=w834, index (row)=0 ("disabled index (col)")) -> (element=→"SCAN OP60":string[])  [unwired: 1 in]
                n334 = call "RESPONSE_LOGIC.vi"("Array"=w834) -> ("Not Found"=w832:i32[])  [unwired: 10 in]
                "OP60 STATUS" <- w832
                n335 = call "PADMINI_AUTO_BARCODE_STATUS 60.vi"("Enum"=enum16{"Read", "Write"}."Write", "error in (no error)"=w848, "I/P"=w832) -> ("error out"=w847:errorcluster)  [unwired: 7 in, 1 out]
              }
              frame True {
                w853 = i32[] [0, 0, 0, 0, 0]  # I/P
                n336 = call "PADMINI_AUTO_BARCODE_STATUS 60.vi"("Enum"=enum16{"Read", "Write"}."Write", "error in (no error)"=w857, "I/P"=w853) -> ("error out"=w856:errorcluster)  [unwired: 7 in, 1 out]
              }
            }
            n337 = flat-sequence {
              tunnel: [w860] -> w825
              tunnel: w826 -> [w860]
              frame #0 {
                # "UPDATE op 60 SCAN sTATUS"
                n338 = global write "DATA LOG.vi" "OP 60 Outputs"(TRUE) -> ()
              }
            }
          }
          frame "DATALOG6" {
            w874 = T17 2 items=["no dialog", "OK message", "continue or stop message", "OK message + warnings", "continue/stop + warnings"] ("type of dialog (OK msg:1)")
            # "datalog of OP 60"
            n339 = call "PADMINI_AUTO_BARCODE_STRING 60.vi"("Enum"=enum16{"Read", "Write"}."Read", "error in (no error)"=w866) -> ("error out"=w868:errorcluster, "Input 2"=w862:string[])  [unwired: 8 in]
            n340 = call "PADMINI_AUTO_CYCLE VALUE 60.vi"("Enum"=enum16{"Read", "Write"}."Read", "error in (no error)"=w866) -> ("Input 2"=w864:sgl[])  [unwired: 8 in, 1 out]
            n341 = Number To Fractional String(number=w864, precision (6)=i16 2) -> (F-format string=w863:string[])  [unwired: 2 in]
            n342 = case shown="False" w879 {
              tunnel: w880 -> [w907 w935]
              tunnel: w868 -> [w908 w934]
              tunnel: [w911 w933] -> w877
              tunnel: [w910 w932] -> w875
              tunnel: w878 -> [w906 _]
              tunnel: w863 -> [w902 w915]
              tunnel: w862 -> [w898 w914]
              frame False {
                # "DO TRACEBILITY"
                n343 = Index Array(array=w898) -> (element #1=w899:string, element #2=w890:string, element #3=w889:string, element #4=w888:string, element #5=w887:string, element #6=w886:string, element #7=w885:string, element #8=w884:string)  [unwired: 8 in]
                n344 = local read "SHIFT"() -> (w909:string)
                n345 = Index Array(array=w902) -> (element #1=w896:string, element #2=w895:string, element #3=w894:string, element #4=w893:string, element #5=w892:string, element #6=w891:string)  [unwired: 6 in]
                n346 = call <vilib>:"Trim Whitespace.vi"("string"=w899) -> ("trimmed string"=w900:string)  [unwired: 1 in]
                n347 = call "PADMINI_SHIFT_DATE.vi"("SHIFT"=w909) -> ("date/time string"=w897:string)  [unwired: 10 in]
                n348 = Format Into String(format string="Where BARCODE='%s' ", w900) -> (resulting string=w904:string)  [unwired: 2 in, 1 out]
                n349 = Bundle("date/time string"=w897, "Input 2"=w896, "Input 2"=w890, "Input 2"=w895, "Input 2"=w889, "Input 2"=w894, "Input 2"=w888, "Input 2"=w893, "Input 2"=w887, "Input 2"=w892, "Input 2"=w886, "Input 2"=w891, "Input 2"=w885, "Input 2"=w884) -> (w901:T27)  [unwired: 1 in]
                n350 = call <vilib>:"DB Tools Update Data.vi"("condition"=w904, "data"=w901, "error in (no error)"=w908, "columns"=string[] ["OP60_DATE", "OP60_SCREW1_DATA_Nm", "OP60_SCREW1_STATUS", "OP60_SCREW2_DATA_Nm", "OP60_SCREW2_STATUS", "OP60_SCREW3_DATA_Nm", "OP60_SCREW3_STATUS", "OP60_SCREW4_DATA_Nm", "OP60_SCREW4_STATUS", "OP60_SCREW5_DATA_Nm", "OP60_SCREW5_STATUS", "OP60_SCREW6_DATA_Nm", "OP60_SCREW6_STATUS", "OP60_FINAL_RESULT"], "table"=w906, "connection reference"=w907) -> ("error out"=w910:errorcluster, "connection reference out"=w911:T16)  [unwired: 4 in]
              }
              frame True {
                # "TRAC BYPASS"
                n351 = local read "SHIFT"() -> (w912:string)
                n352 = call "PADMINI_SHIFT_DATE.vi"("SHIFT"=w912) -> ("date/time string"=w913:string)  [unwired: 10 in]
                n353 = Index Array(array=w914) -> (element #2=w923:string, element #3=w922:string, element #4=w921:string, element #5=w919:string, element #6=w927:string, element #7=w928:string)  [unwired: 7 in, 1 out]
                n354 = Index Array(array=w915) -> (element #1=w926:string, element #2=w925:string, element #3=w924:string, element #4=w920:string, element #5=w918:string, element #6=w917:string)  [unwired: 6 in]
                n355 = Bundle("date/time string"=w913, "SHIFT"=w912, "Input 2"=w926, "Input 2"=w923, "Input 2"=w925, "Input 2"=w922, "Input 2"=w924, "Input 2"=w921, "Input 2"=w920, "Input 2"=w919, "Input 2"=w918, "Input 2"=w917, "Input 2"=w927, "Input 2"=w928) -> (w916:T28)  [unwired: 1 in]
                n356 = To Variant(anything=w916) -> (Variant=w931:variant)
                n357 = call <vilib>:"DB Tools Insert Data.vi"("data"=w931, "error in (no error)"=w934, "columns"=string[] ["DATE", "SHIFT", "ST6_SCREW1_DATA", "ST6_SCREW1_STATUS", "ST6_SCREW2_DATA", "ST6_SCREW2_STATUS", "ST6_SCREW3_DATA", "ST6_SCREW3_STATUS", "ST6_SCREW4_DATA", "ST6_SCREW4_STATUS", "ST6_SCREW5_DATA", "ST6_SCREW5_STATUS", "ST6_SCREW6_DATA", "ST6_SCREW6_STATUS", "ST6_FINAL_RST"], "table"="ST6_REPORT", "connection reference"=w935) -> ("error out"=w932:errorcluster, "connection reference out"=w933:T16)  [unwired: 5 in]
              }
            }
            n358 = call <vilib>:"Simple Error Handler.vi"("type of dialog (OK msg:1)"=w874, "error in (no error)"=w875) -> ("error out"=w873:errorcluster)  [unwired: 3 in, 4 out]
            n359 = call <vilib>:"Clear Errors.vi"("error in (no error)"=w873) -> ("error out"=w871:errorcluster)  [unwired: 5 in, 1 out]
            n360 = flat-sequence {
              tunnel: [w883] -> w861
              tunnel: w871 -> [w883]
              frame #0 {
                # "UPDATE op 20 save"
                n361 = global write "DATA LOG.vi" "OP 60 reset"(TRUE) -> ()
              }
            }
          }
          frame "SCAN7" {
            # "STATION OP 70"
            n362 = case shown="False" w942 {
              tunnel: w946 -> [w967 w973]
              tunnel: w945 -> [w960 w972]
              tunnel: w944 -> [w952 _]
              tunnel: [w962 w971] -> w941
              tunnel: [w961 w973] -> w943
              tunnel: [w953 "" ("trimmed string")] -> _
              frame False {
                n363 = call "PADMINI_AUTO_BARCODE_STRING 70.vi"("Enum"=enum16{"Read", "Write"}."Read", "error in (no error)"=w960) -> ("error out"=w959:errorcluster, "Input 2"=w955:string[])  [unwired: 8 in]
                n364 = Index Array(array=w955) -> (element=w954:string)  [unwired: 1 in]
                n365 = call <vilib>:"Trim Whitespace.vi"("string"=w954) -> ("trimmed string"=w953:string)  [unwired: 1 in]
                n366 = Format Into String(format string="WHERE BARCODE  ='%s'", w953) -> (resulting string=w956:string)  [unwired: 2 in, 1 out]
                n367 = call <vilib>:"DB Tools Select Data.vi"("condition"=w956, "error in (no error)"=w959, "columns"=string[] ["BARCODE", "OP60_FINAL_RESULT", "OP70_FINAL_RESULT"], "table"=w952, "connection reference"=w967) -> ("error out"=w965:errorcluster, "data"=w964:variant[][], "connection reference out"=w961:T16)  [unwired: 1 in]
                n368 = call "PADMINI_varient_to_data.vi"("error in (no error)"=w965, "data"=w964) -> ("error out"=w963:errorcluster, "Array"=w949:string[][])  [unwired: 8 in]
                n369 = Index Array(array=w949, index (row)=0 ("disabled index (col)")) -> (element=→"SCAN OP70":string[])  [unwired: 1 in]
                n370 = call "RESPONSE_LOGIC.vi"("Array"=w949) -> ("Not Found"=w947:i32[])  [unwired: 10 in]
                "OP70 STATUS" <- w947
                n371 = call "PADMINI_AUTO_BARCODE_STATUS 70.vi"("Enum"=enum16{"Read", "Write"}."Write", "error in (no error)"=w963, "I/P"=w947) -> ("error out"=w962:errorcluster)  [unwired: 7 in, 1 out]
              }
              frame True {
                w968 = i32[] [0, 0, 0, 0, 0]  # I/P
                n372 = call "PADMINI_AUTO_BARCODE_STATUS 70.vi"("Enum"=enum16{"Read", "Write"}."Write", "error in (no error)"=w972, "I/P"=w968) -> ("error out"=w971:errorcluster)  [unwired: 7 in, 1 out]
              }
            }
            n373 = flat-sequence {
              tunnel: [w975] -> w940
              tunnel: w941 -> [w975]
              frame #0 {
                # "UPDATE op 70 SCAN sTATUS"
                n374 = global write "DATA LOG.vi" "OP 70 Outputs"(TRUE) -> ()
              }
            }
          }
          frame "DATALOG7" {
            # "datalog of OP 70"
            n375 = call "PADMINI_AUTO_BARCODE_STRING 70.vi"("Enum"=enum16{"Read", "Write"}."Read", "error in (no error)"=w981) -> ("error out"=w983:errorcluster, "Input 2"=w977:string[])  [unwired: 8 in]
            n376 = call "PADMINI_AUTO_CYCLE VALUE 70.vi"("Enum"=enum16{"Read", "Write"}."Read", "error in (no error)"=w981) -> ("Input 2"=w979:sgl[])  [unwired: 8 in, 1 out]
            n377 = Number To Fractional String(number=w979, precision (6)=i16 4) -> (F-format string=w978:string[])  [unwired: 2 in]
            n378 = case shown="False" w991 {
              tunnel: w992 -> [w1010 w1028]
              tunnel: w983 -> [w1011 w1027]
              tunnel: [w1013 w1026] -> w989
              tunnel: [w1012 w1025] -> w987
              tunnel: w990 -> [w1009 _]
              tunnel: w978 -> [w1005 w1015]
              tunnel: w977 -> [w1000 w1014]
              frame False {
                # "DO TRACEBILITY"
                n379 = Index Array(array=w1000) -> (element #1=w1001:string, element #2=w999:string)  [unwired: 2 in]
                n380 = call <vilib>:"Trim Whitespace.vi"("string"=w1001) -> ("trimmed string"=w1002:string)  [unwired: 1 in]
                n381 = local read "SHIFT"() -> (w997:string)
                n382 = Index Array(array=w1005) -> (element #1=w1004:string, element #2=w998:string)  [unwired: 2 in]
                n383 = call "PADMINI_SHIFT_DATE.vi"("SHIFT"=w997) -> ("date/time string"=w996:string)  [unwired: 10 in]
                n384 = Bundle("date/time string"=w996, "Input 2"=w1004, "Input 2"=w998, "Input 2"=w999) -> (w1003:T29)  [unwired: 1 in]
                n385 = Format Into String(format string="Where BARCODE='%s' ", w1002) -> (resulting string=w1007:string)  [unwired: 2 in, 1 out]
                n386 = call <vilib>:"DB Tools Update Data.vi"("condition"=w1007, "data"=w1003, "error in (no error)"=w1011, "columns"=string[] ["OP70_DATE", "OP70_FULL_OPEN", "OP70_FULL_CLOSE", "OP70_FINAL_RESULT"], "table"=w1009, "connection reference"=w1010) -> ("error out"=w1012:errorcluster, "connection reference out"=w1013:T16)  [unwired: 4 in]
              }
              frame True {
                # "TRAC BYPASS"
                n387 = local read "SHIFT"() -> (w1016:string)
                n388 = call "PADMINI_SHIFT_DATE.vi"("SHIFT"=w1016) -> ("date/time string"=w1017:string)  [unwired: 10 in]
                n389 = Index Array(array=w1014) -> (element #2=w1020:string)  [unwired: 2 in, 1 out]
                n390 = Index Array(array=w1015) -> (element #1=w1021:string, element #2=w1019:string)  [unwired: 2 in]
                n391 = Bundle("date/time string"=w1017, "SHIFT"=w1016, "Input 2"=w1021, "Input 2"=w1019, "Input 2"=w1020) -> (w1018:T30)  [unwired: 1 in]
                n392 = To Variant(anything=w1018) -> (Variant=w1024:variant)
                n393 = call <vilib>:"DB Tools Insert Data.vi"("data"=w1024, "error in (no error)"=w1027, "columns"=string[] ["DATE_OP70", "SHIFT", "OP70_FULL_OPEN", "OP70_FULL_CLOSE", "OP70_FINAL_RST"], "table"="ST7_REPORT", "connection reference"=w1028) -> ("error out"=w1025:errorcluster, "connection reference out"=w1026:T16)  [unwired: 5 in]
              }
            }
            n394 = flat-sequence {
              tunnel: [w995] -> w976
              tunnel: w987 -> [w995]
              frame #0 {
                # "UPDATE op 20 save"
                n395 = global write "DATA LOG.vi" "OP 70 reset"(TRUE) -> ()
              }
            }
          }
          frame "SCAN8" {
            # "STATION OP 80"
            n396 = case shown="False" w1035 {
              tunnel: w1039 -> [w1060 w1066]
              tunnel: w1038 -> [w1053 w1065]
              tunnel: w1037 -> [w1045 _]
              tunnel: [w1055 w1064] -> w1034
              tunnel: [w1054 w1066] -> w1036
              tunnel: [w1046 "" ("trimmed string")] -> _
              frame False {
                (unwired) "REPORT"
                n397 = call "PADMINI_AUTO_BARCODE_STRING 80.vi"("Enum"=enum16{"Read", "Write"}."Read", "error in (no error)"=w1053) -> ("error out"=w1052:errorcluster, "Input 2"=w1048:string[])  [unwired: 8 in]
                n398 = Index Array(array=w1048) -> (element=w1047:string)  [unwired: 1 in]
                n399 = call <vilib>:"Trim Whitespace.vi"("string"=w1047) -> ("trimmed string"=w1046:string)  [unwired: 1 in]
                n400 = Format Into String(format string="WHERE BARCODE  ='%s'", w1046) -> (resulting string=w1049:string)  [unwired: 2 in, 1 out]
                n401 = call <vilib>:"DB Tools Select Data.vi"("condition"=w1049, "error in (no error)"=w1052, "columns"=string[] ["BARCODE", "OP70_FINAL_RESULT", "OP80_FINAL_RESULT"], "table"=w1045, "connection reference"=w1060) -> ("error out"=w1058:errorcluster, "data"=w1057:variant[][], "connection reference out"=w1054:T16)  [unwired: 1 in]
                n402 = call "PADMINI_varient_to_data.vi"("error in (no error)"=w1058, "data"=w1057) -> ("error out"=w1056:errorcluster, "Array"=w1042:string[][])  [unwired: 8 in]
                n403 = Index Array(array=w1042, index (row)=0 ("disabled index (col)")) -> (element=→"SCAN OP80":string[])  [unwired: 1 in]
                n404 = call "RESPONSE_LOGIC.vi"("Array"=w1042) -> ("Not Found"=w1041:i32[])  [unwired: 10 in]
                "OP80 STATUS" <- w1041
                n405 = call "PADMINI_AUTO_BARCODE_STATUS 80.vi"("Enum"=enum16{"Read", "Write"}."Write", "error in (no error)"=w1056, "I/P"=w1041) -> ("error out"=w1055:errorcluster)  [unwired: 7 in, 1 out]
              }
              frame True {
                w1061 = i32[] [0, 0, 0, 0, 0]  # I/P
                n406 = call "PADMINI_AUTO_BARCODE_STATUS 80.vi"("Enum"=enum16{"Read", "Write"}."Write", "error in (no error)"=w1065, "I/P"=w1061) -> ("error out"=w1064:errorcluster)  [unwired: 7 in, 1 out]
              }
            }
            n407 = flat-sequence {
              tunnel: [w1068] -> w1033
              tunnel: w1034 -> [w1068]
              frame #0 {
                # "UPDATE op 80 SCAN sTATUS"
                n408 = global write "DATA LOG.vi" "OP 80 Outputs"(TRUE) -> ()
              }
            }
          }
          frame "DATALOG8" {
            w1083 = T17 2 items=["no dialog", "OK message", "continue or stop message", "OK message + warnings", "continue/stop + warnings"] ("type of dialog (OK msg:1)")
            # "datalog of OP 80"
            n409 = call "PADMINI_AUTO_BARCODE_STRING 80.vi"("Enum"=enum16{"Read", "Write"}."Read", "error in (no error)"=w1075) -> ("error out"=w1077:errorcluster, "Input 2"=w1071:string[])  [unwired: 8 in]
            n410 = call "PADMINI_AUTO_CYCLE VALUE 80.vi"("Enum"=enum16{"Read", "Write"}."Read", "error in (no error)"=w1075) -> ("Input 2"=w1073:sgl[])  [unwired: 8 in, 1 out]
            n411 = Number To Fractional String(number=w1073, precision (6)=i16 2) -> (F-format string=w1072:string[])  [unwired: 2 in]
            n412 = case shown="True" w1069 {
              tunnel: w1088 -> [w1106 w1125]
              tunnel: w1077 -> [w1107 w1124]
              tunnel: [w1109 w1123] -> w1086
              tunnel: [w1108 w1122] -> w1084
              tunnel: w1087 -> [w1105 w1110]
              tunnel: w1072 -> [w1101 w1115]
              tunnel: w1071 -> [w1097 w1116]
              frame False {
                # "DO TRACEBILITY"
                n413 = Index Array(array=w1097) -> (element #1=w1098:string, element #2=w1093:string, element #3=w1092:string)  [unwired: 3 in]
                n414 = call <vilib>:"Trim Whitespace.vi"("string"=w1098) -> ("trimmed string"=w1099:string)  [unwired: 1 in]
                n415 = local read "SHIFT"() -> (w1096:string)
                n416 = Index Array(array=w1101) -> (element=w1094:string)  [unwired: 1 in]
                n417 = call "PADMINI_SHIFT_DATE.vi"("SHIFT"=w1096) -> ("date/time string"=w1095:string)  [unwired: 10 in]
                n418 = Bundle("date/time string"=w1095, "Input 2"=w1093, "Input 2"=w1094, "Input 2"=w1092) -> (w1100:T29)  [unwired: 1 in]
                n419 = Format Into String(format string="Where BARCODE='%s' ", w1099) -> (resulting string=w1103:string)  [unwired: 2 in, 1 out]
                n420 = call <vilib>:"DB Tools Update Data.vi"("condition"=w1103, "data"=w1100, "error in (no error)"=w1107, "columns"=string[] ["OP80_DATE", "OP80_LOCTITE_STATUS", "OP80_PLUG_PRESS_LOAD_kg", "OP80_FINAL_RESULT"], "table"=w1105, "connection reference"=w1106) -> ("error out"=w1108:errorcluster, "connection reference out"=w1109:T16)  [unwired: 4 in]
              }
              frame True {
                (unwired) "ST8_REPORT"
                # "TRAC BYPASS"
                n421 = local read "SHIFT"() -> (w1112:string)
                n422 = call "PADMINI_SHIFT_DATE.vi"("SHIFT"=w1112) -> ("date/time string"=w1111:string)  [unwired: 10 in]
                n423 = Index Array(array=w1116) -> (element #1=w1113:string, element #2=w1120:string, element #3=w1119:string)  [unwired: 3 in]
                n424 = Index Array(array=w1115) -> (element=w1118:string)  [unwired: 1 in]
                n425 = Bundle("Input 2"=w1113, "SHIFT"=w1112, "date/time string"=w1111, "Input 2"=w1118, "Input 2"=w1120, "Input 2"=w1119) -> (w1117:T31)  [unwired: 1 in]
                n426 = To Variant(anything=w1117) -> (Variant=w1121:variant)
                n427 = call <vilib>:"DB Tools Insert Data.vi"("data"=w1121, "error in (no error)"=w1124, "columns"=string[] ["BARCODE", "SHIFT", "OP80_DATE", "OP80_LOCTITE_STATUS", "OP80_PLUG_PRESS_LOAD_kg", "OP80_FINAL_RESULT"], "table"=w1110, "connection reference"=w1125) -> ("error out"=w1122:errorcluster, "connection reference out"=w1123:T16)  [unwired: 5 in]
              }
            }
            n428 = call <vilib>:"Simple Error Handler.vi"("type of dialog (OK msg:1)"=w1083, "error in (no error)"=w1084) -> ("error out"=w1082:errorcluster)  [unwired: 3 in, 4 out]
            n429 = call <vilib>:"Clear Errors.vi"("error in (no error)"=w1082) -> ("error out"=w1080:errorcluster)  [unwired: 5 in, 1 out]
            n430 = flat-sequence {
              tunnel: [w1091] -> w1070
              tunnel: w1080 -> [w1091]
              frame #0 {
                # "UPDATE op 20 save"
                n431 = global write "DATA LOG.vi" "OP 80 reset"(TRUE) -> ()
              }
            }
          }
          frame "SCAN9" {
            # "STATION OP 90"
            n432 = case shown="False" w1132 {
              tunnel: w1136 -> [w1157 w1163]
              tunnel: w1135 -> [w1150 w1162]
              tunnel: w1134 -> [w1142 _]
              tunnel: [w1152 w1161] -> w1131
              tunnel: [w1151 w1163] -> w1133
              tunnel: [w1143 "" ("trimmed string")] -> _
              frame False {
                (unwired) "REPORT"
                n433 = call "PADMINI_AUTO_BARCODE_STRING 90.vi"("Enum"=enum16{"Read", "Write"}."Read", "error in (no error)"=w1150) -> ("error out"=w1149:errorcluster, "Input 2"=w1145:string[])  [unwired: 8 in]
                n434 = Index Array(array=w1145) -> (element=w1144:string)  [unwired: 1 in]
                n435 = call <vilib>:"Trim Whitespace.vi"("string"=w1144) -> ("trimmed string"=w1143:string)  [unwired: 1 in]
                n436 = Format Into String(format string="WHERE BARCODE  ='%s'", w1143) -> (resulting string=w1146:string)  [unwired: 2 in, 1 out]
                n437 = call <vilib>:"DB Tools Select Data.vi"("condition"=w1146, "error in (no error)"=w1149, "columns"=string[] ["BARCODE", "OP80_FINAL_RESULT", "OP90_FINAL_RESULT"], "table"=w1142, "connection reference"=w1157) -> ("error out"=w1155:errorcluster, "data"=w1154:variant[][], "connection reference out"=w1151:T16)  [unwired: 1 in]
                n438 = call "PADMINI_varient_to_data.vi"("error in (no error)"=w1155, "data"=w1154) -> ("error out"=w1153:errorcluster, "Array"=w1139:string[][])  [unwired: 8 in]
                n439 = Index Array(array=w1139, index (row)=0 ("disabled index (col)")) -> (element=→"SCAN OP90":string[])  [unwired: 1 in]
                n440 = call "RESPONSE_LOGIC.vi"("Array"=w1139) -> ("Not Found"=w1137:i32[])  [unwired: 10 in]
                "OP90 STATUS" <- w1137
                n441 = call "PADMINI_AUTO_BARCODE_STATUS 90.vi"("Enum"=enum16{"Read", "Write"}."Write", "error in (no error)"=w1153, "I/P"=w1137) -> ("error out"=w1152:errorcluster)  [unwired: 7 in, 1 out]
              }
              frame True {
                w1158 = i32[] [0, 0, 0, 0, 0]  # I/P
                n442 = call "PADMINI_AUTO_BARCODE_STATUS 90.vi"("Enum"=enum16{"Read", "Write"}."Write", "error in (no error)"=w1162, "I/P"=w1158) -> ("error out"=w1161:errorcluster)  [unwired: 7 in, 1 out]
              }
            }
            n443 = flat-sequence {
              tunnel: [w1165] -> w1130
              tunnel: w1131 -> [w1165]
              frame #0 {
                # "UPDATE op 90 SCAN sTATUS"
                n444 = global write "DATA LOG.vi" "OP 90 Outputs"(TRUE) -> ()
              }
            }
          }
          frame "DATALOG9" {
            w1179 = T17 2 items=["no dialog", "OK message", "continue or stop message", "OK message + warnings", "continue/stop + warnings"] ("type of dialog (OK msg:1)")
            # "datalog of OP 90"
            n445 = call "PADMINI_AUTO_BARCODE_STRING 90.vi"("Enum"=enum16{"Read", "Write"}."Read", "error in (no error)"=w1171) -> ("error out"=w1173:errorcluster, "Input 2"=w1168:string[])  [unwired: 8 in]
            n446 = call "PADMINI_AUTO_CYCLE VALUE 90.vi"("Enum"=enum16{"Read", "Write"}."Read", "error in (no error)"=w1171) -> ("Input 2"=w1167:sgl[])  [unwired: 8 in, 1 out]
            n447 = Number To Fractional String(number=w1167, precision (6)=i16 2) -> (F-format string=w1169:string[])  [unwired: 2 in]
            n448 = case shown="False" w1184 {
              tunnel: w1185 -> [w1204 w1223]
              tunnel: w1173 -> [w1205 w1222]
              tunnel: [w1207 w1221] -> w1182
              tunnel: [w1206 w1220] -> w1180
              tunnel: w1183 -> [w1203 _]
              tunnel: w1169 -> [w1199 w1212]
              tunnel: w1168 -> [w1195 w1211]
              frame False {
                # "DO TRACEBILITY"
                n449 = Index Array(array=w1195) -> (element #1=w1196:string, element #2=w1193:string, element #3=w1191:string)  [unwired: 3 in]
                n450 = call <vilib>:"Trim Whitespace.vi"("string"=w1196) -> ("trimmed string"=w1197:string)  [unwired: 1 in]
                n451 = local read "SHIFT"() -> (w1190:string)
                n452 = Index Array(array=w1199) -> (element #1=w1194:string, element #2=w1192:string)  [unwired: 2 in]
                n453 = call "PADMINI_SHIFT_DATE.vi"("SHIFT"=w1190) -> ("date/time string"=w1189:string)  [unwired: 10 in]
                n454 = Bundle("date/time string"=w1189, "Input 2"=w1194, "Input 2"=w1193, "Input 2"=w1192, "Input 2"=w1191) -> (w1198:T22)  [unwired: 1 in]
                n455 = Format Into String(format string="Where BARCODE='%s' ", w1197) -> (resulting string=w1201:string)  [unwired: 2 in, 1 out]
                n456 = call <vilib>:"DB Tools Update Data.vi"("condition"=w1201, "data"=w1198, "error in (no error)"=w1205, "columns"=string[] ["OP90_DATE", "OP90_SEAT_LEAK_LP", "OP90_SEAT_STATUS", "OP90_STEAM_LEAK_sccm", "OP90_FINAL_RESULT"], "table"=w1203, "connection reference"=w1204) -> ("error out"=w1206:errorcluster, "connection reference out"=w1207:T16)  [unwired: 4 in]
              }
              frame True {
                # "TRAC BYPASS"
                n457 = local read "SHIFT"() -> (w1208:string)
                n458 = call "PADMINI_SHIFT_DATE.vi"("SHIFT"=w1208) -> ("date/time string"=w1209:string)  [unwired: 10 in]
                n459 = Index Array(array=w1211) -> (element #2=w1216:string, element #3=w1214:string)  [unwired: 3 in, 1 out]
                n460 = Index Array(array=w1212) -> (element #1=w1217:string, element #2=w1215:string)  [unwired: 2 in]
                n461 = Bundle("date/time string"=w1209, "SHIFT"=w1208, "Input 2"=w1217, "Input 2"=w1216, "Input 2"=w1215, "Input 2"=w1214) -> (w1213:T23)  [unwired: 1 in]
                n462 = To Variant(anything=w1213) -> (Variant=w1219:variant)
                n463 = call <vilib>:"DB Tools Insert Data.vi"("data"=w1219, "error in (no error)"=w1222, "columns"=string[] ["DATE", "SHIFT", "ST9_SEAT_LT_DATA", "ST9_SEAT_STATUS", "ST9_STEAM_LT_DATA", "ST9_FINAL_RST"], "table"="ST9_REPORT", "connection reference"=w1223) -> ("error out"=w1220:errorcluster, "connection reference out"=w1221:T16)  [unwired: 5 in]
              }
            }
            n464 = call <vilib>:"Simple Error Handler.vi"("type of dialog (OK msg:1)"=w1179, "error in (no error)"=w1180) -> ("error out"=w1178:errorcluster)  [unwired: 3 in, 4 out]
            n465 = call <vilib>:"Clear Errors.vi"("error in (no error)"=w1178) -> ("error out"=w1176:errorcluster)  [unwired: 5 in, 1 out]
            n466 = flat-sequence {
              tunnel: [w1188] -> w1166
              tunnel: w1176 -> [w1188]
              frame #0 {
                # "UPDATE op 20 save"
                n467 = global write "DATA LOG.vi" "OP 90 reset"(TRUE) -> ()
              }
            }
          }
          frame "SCAN10" {
            # "STATION OP 10"
            n468 = case shown="False" w1230 {
              tunnel: w1234 -> [w1255 w1261]
              tunnel: w1233 -> [w1249 w1260]
              tunnel: w1232 -> [w1241 _]
              tunnel: [w1239 w1259] -> w1229
              tunnel: [w1250 w1261] -> w1231
              tunnel: [w1242 "" ("trimmed string")] -> _
              frame False {
                (unwired) "REPORT"
                n469 = call "PADMINI_AUTO_BARCODE_STRING 100.vi"("Enum"=enum16{"Read", "Write"}."Read", "error in (no error)"=w1249) -> ("error out"=w1248:errorcluster, "Input 2"=w1244:string[])  [unwired: 8 in]
                n470 = Index Array(array=w1244) -> (element=w1243:string)  [unwired: 1 in]
                n471 = call <vilib>:"Trim Whitespace.vi"("string"=w1243) -> ("trimmed string"=w1242:string)  [unwired: 1 in]
                n472 = Format Into String(format string="WHERE BARCODE  ='%s'", w1242) -> (resulting string=w1245:string)  [unwired: 2 in, 1 out]
                n473 = call <vilib>:"DB Tools Select Data.vi"("condition"=w1245, "error in (no error)"=w1248, "columns"=string[] ["BARCODE", "OP90_FINAL_RESULT", "OP100_FINAL_RESULT"], "table"=w1241, "connection reference"=w1255) -> ("error out"=w1253:errorcluster, "data"=w1252:variant[][], "connection reference out"=w1250:T16)  [unwired: 1 in]
                n474 = call "PADMINI_varient_to_data.vi"("error in (no error)"=w1253, "data"=w1252) -> ("error out"=w1251:errorcluster, "Array"=w1237:string[][])  [unwired: 8 in]
                n475 = Index Array(array=w1237, index (row)=0 ("disabled index (col)")) -> (element=→"SCAN OP100":string[])  [unwired: 1 in]
                n476 = call "RESPONSE_LOGIC.vi"("Array"=w1237) -> ("Not Found"=w1235:i32[])  [unwired: 10 in]
                "OP100 STATUS" <- w1235
                n477 = call "PADMINI_AUTO_BARCODE_STATUS 100.vi"("Enum"=enum16{"Read", "Write"}."Write", "error in (no error)"=w1251, "I/P"=w1235) -> ("error out"=w1239:errorcluster)  [unwired: 7 in, 1 out]
              }
              frame True {
                w1256 = i32[] [0, 0, 0, 0, 0]  # I/P
                n478 = call "PADMINI_AUTO_BARCODE_STATUS 100.vi"("Enum"=enum16{"Read", "Write"}."Write", "error in (no error)"=w1260, "I/P"=w1256) -> ("error out"=w1259:errorcluster)  [unwired: 7 in, 1 out]
              }
            }
            n479 = flat-sequence {
              tunnel: [w1263] -> w1228
              tunnel: w1229 -> [w1263]
              frame #0 {
                # "UPDATE op 100 SCAN sTATUS"
                n480 = global write "DATA LOG.vi" "OP 100 Outputs"(TRUE) -> ()
              }
            }
          }
          frame "SCAN11" {
            # "STATION OP 110"
            n481 = case shown="False" w1270 {
              tunnel: w1274 -> [w1307 w1332]
              tunnel: w1273 -> [w1281 w1331]
              tunnel: w1272 -> [w1284 _]
              tunnel: [w1304 w1330] -> w1269
              tunnel: [w1286 w1332] -> w1271
              frame False {
                (unwired) "P5314216;S07122024020102;VA1105000100"
                # "OP100 OK\nOP 100 NG"
                n482 = call "PADMINI_AUTO_BARCODE_STRING 110.vi"("Enum"=enum16{"Read", "Write"}."Read", "error in (no error)"=w1281) -> ("error out"=w1282:errorcluster, "Input 2"=w1280:string[])  [unwired: 8 in]
                n483 = Index Array(array=w1280) -> (element=w1301:string)  [unwired: 1 in]
                n484 = call <vilib>:"Trim Whitespace.vi"("string"=w1301) -> ("trimmed string"=w1278:string)  [unwired: 1 in]
                n485 = call "String_Conversion_OP110.vi"("String in"=w1278) -> ("String out"=w1279:string)  [unwired: 9 in, 1 out]
                n486 = Format Into String(format string="WHERE BARCODE  ='%s'", w1279) -> (resulting string=w1285:string)  [unwired: 2 in, 1 out]
                "resulting string" <- w1285
                n487 = call <vilib>:"DB Tools Select Data.vi"("condition"=w1285, "error in (no error)"=w1282, "columns"=string[] ["BARCODE", "OP100_FINAL_RESULT", "OP110_BIN_NO"], "table"=w1284, "connection reference"=w1307) -> ("error out"=w1306:errorcluster, "data"=w1305:variant[][], "connection reference out"=w1287:T16)  [unwired: 1 in]
                n488 = call "PADMINI_varient_to_data.vi"("error in (no error)"=w1306, "data"=w1305) -> ("error out"=w1288:errorcluster, "Array"=w1292:string[][])  [unwired: 8 in]
                n489 = Index Array(array=w1292, index (row)=0 ("disabled index (col)")) -> (element=w1291:string[])  [unwired: 1 in]
                "SCAN OP110" <- w1291
                n490 = Index Array(array=w1291) -> (element #1=w1299:string, element #2=w1296:string, element #3=w1276:string)  [unwired: 3 in]
                n491 = Equal?(x=w1276, y="") -> (x = y?=w1275:bool)
                n492 = Equal?(x="", y=w1299) -> (x = y?=w1298:bool)
                n493 = Equal?(x=w1296, y="OK") -> (x = y?=w1297:bool)
                n494 = case shown="False" w1298 {
                  tunnel: w1297 -> [w1314 _]
                  tunnel: [w1315 w1327] -> w1290
                  tunnel: [w1313 w1326] -> w1289
                  tunnel: w1288 -> [w1312 w1326]
                  tunnel: w1287 -> [w1311 w1325]
                  tunnel: [w1310 w1325] -> w1286
                  tunnel: w1284 -> [w1309 _]
                  tunnel: w1275 -> [w1308 _]
                  frame False {
                    # "BARCODE FOUND"
                    n495 = case shown="True" w1314 {
                      tunnel: [w1318 w1320] -> w1315
                      tunnel: [w1317 w1324] -> w1313
                      tunnel: w1312 -> [w1317 w1324]
                      tunnel: w1311 -> [w1316 w1323]
                      tunnel: [w1316 w1323] -> w1310
                      tunnel: w1309 -> [_ _]
                      tunnel: w1308 -> [_ w1322]
                      frame False {
                        w1318 = i32[] [0, 1, 0]  # OK
                        # "CT ST REPEAT NG & EMPTY"
                      }
                      frame True {
                        w1319 = i32[] [1, 0, 1]  # OK but repeat
                        w1321 = i32[] [1, 0, 0]  # OK and not repeat
                        # "CT ST REPEAT EMPTY"
                        n496 = Select(t=w1321, s=w1322, f=w1319) -> (s? t:f=w1320:i32[])
                      }
                    }
                  }
                  frame True {
                    w1327 = i32[] [0, 1, 0]  # Not Found
                    # "nO BARCODE FOUND"
                  }
                }
                "OP110 STATUS" <- w1290
                n497 = call "PADMINI_AUTO_BARCODE_STATUS 110.vi"("Enum"=enum16{"Read", "Write"}."Write", "error in (no error)"=w1289, "I/P"=w1290) -> ("error out"=w1304:errorcluster)  [unwired: 7 in, 1 out]
              }
              frame True {
                w1328 = i32[] [0, 0, 0, 0, 0]  # I/P
                n498 = call "PADMINI_AUTO_BARCODE_STATUS 100.vi"("Enum"=enum16{"Read", "Write"}."Write", "error in (no error)"=w1331, "I/P"=w1328) -> ("error out"=w1330:errorcluster)  [unwired: 7 in, 1 out]
              }
            }
            n499 = flat-sequence {
              tunnel: [w1334] -> w1268
              tunnel: w1269 -> [w1334]
              frame #0 {
                # "UPDATE op 100 SCAN sTATUS"
                n500 = global write "DATA LOG.vi" "OP 110 Outputs"(TRUE) -> ()
              }
            }
          }
          frame "DATALOG10" {
            w1348 = T17 2 items=["no dialog", "OK message", "continue or stop message", "OK message + warnings", "continue/stop + warnings"] ("type of dialog (OK msg:1)")
            # "datalog of OP 100"
            n501 = call "PADMINI_AUTO_BARCODE_STRING 100.vi"("Enum"=enum16{"Read", "Write"}."Read", "error in (no error)"=w1336) -> ("error out"=w1342:errorcluster, "Input 2"=w1338:string[])  [unwired: 8 in]
            n502 = call "PADMINI_AUTO_CYCLE VALUE 100.vi"("Enum"=enum16{"Read", "Write"}."Read", "error in (no error)"=w1336) -> ("Input 2"=w1337:sgl[])  [unwired: 8 in, 1 out]
            n503 = Number To Fractional String(number=w1337, precision (6)=i16 2) -> (F-format string=w1339:string[])  [unwired: 2 in]
            n504 = case shown="False" w1353 {
              tunnel: w1354 -> [w1382 w1407]
              tunnel: w1342 -> [w1383 w1406]
              tunnel: [w1385 w1405] -> w1351
              tunnel: [w1384 w1404] -> w1349
              tunnel: w1352 -> [w1381 _]
              tunnel: w1339 -> [w1377 w1389]
              tunnel: w1338 -> [w1374 w1390]
              frame False {
                # "DO TRACEBILITY"
                n505 = Index Array(array=w1374) -> (element #1=w1373:string, element #2=w1359:string, element #3=w1358:string)  [unwired: 3 in]
                n506 = call <vilib>:"Trim Whitespace.vi"("string"=w1373) -> ("trimmed string"=w1375:string)  [unwired: 1 in]
                n507 = Index Array(array=w1377) -> (element #1=w1370:string, element #2=w1369:string, element #3=w1368:string, element #4=w1367:string, element #5=w1366:string, element #6=w1365:string, element #7=w1364:string, element #8=w1363:string, element #9=w1362:string, element #10=w1361:string, element #11=w1360:string)  [unwired: 11 in]
                n508 = local read "SHIFT"() -> (w1372:string)
                n509 = call "PADMINI_SHIFT_DATE.vi"("SHIFT"=w1372) -> ("date/time string"=w1371:string)  [unwired: 10 in]
                n510 = Bundle("date/time string"=w1371, "Input 2"=w1370, "Input 2"=w1369, "Input 2"=w1368, "Input 2"=w1367, "Input 2"=w1366, "Input 2"=w1365, "Input 2"=w1364, "Input 2"=w1363, "Input 2"=w1362, "Input 2"=w1361, "Input 2"=w1360, "Input 2"=w1359, "Input 2"=w1358) -> (w1376:T27)  [unwired: 1 in]
                n511 = Format Into String(format string="Where BARCODE='%s' ", w1375) -> (resulting string=w1379:string)  [unwired: 2 in, 1 out]
                n512 = call <vilib>:"DB Tools Update Data.vi"("condition"=w1379, "data"=w1376, "error in (no error)"=w1383, "columns"=string[] ["OP100_DATE", "OP100_SENSOR_OP_OPEN_V", "OP100_SENSOR_OP_CLOSE_V", "OP100_SENSOR_OP_FULL_CLOSE_V", "OP100_SENSOR_INITIAL_V", "OP100_MOTOR_START_OF_CLOSE_V", "OP100_MOTOR_FULL_CLOSE_V", "OP100_MOTOR_START_BACK_V", "OP100_MOTOR_FULL_OPEN_V", "OP100_RESPONSE_TIME_FWD_msec", "OP100_RESPONSE_TIME_REV_msec", "OP100_MOTOR_PEAK_CURRENT_A", "OP100_FINAL_RESULT", "OP100_CONNECTOR_CAMERA_STATUS"], "table"=w1381, "connection reference"=w1382) -> ("error out"=w1384:errorcluster, "connection reference out"=w1385:T16)  [unwired: 4 in]
              }
              frame True {
                # "TRAC BYPASS"
                n513 = local read "SHIFT"() -> (w1387:string)
                n514 = Index Array(array=w1390) -> (element=w1394:string)  [unwired: 1 in]
                n515 = call "PADMINI_SHIFT_DATE.vi"("SHIFT"=w1387) -> ("date/time string"=w1388:string)  [unwired: 10 in]
                n516 = Index Array(array=w1389) -> (element #1=w1400:string, element #2=w1399:string, element #3=w1386:string, element #4=w1392:string, element #5=w1398:string, element #6=w1393:string, element #7=w1397:string, element #8=w1396:string, element #9=w1395:string)  [unwired: 9 in]
                n517 = Bundle("date/time string"=w1388, "SHIFT"=w1387, "Input 2"=w1400, "Input 2"=w1399, "Input 2"=w1386, "Input 2"=w1386, "Input 2"=w1386, "Input 2"=w1392, "Input 2"=w1398, "Input 2"=w1393, "Input 2"=w1397, "Input 2"=w1396, "Input 2"=w1395, "Input 2"=w1394) -> (w1391:T28)  [unwired: 1 in]
                n518 = To Variant(anything=w1391) -> (Variant=w1403:variant)
                n519 = call <vilib>:"DB Tools Insert Data.vi"("data"=w1403, "error in (no error)"=w1406, "columns"=string[] ["DATE", "SHIFT", "ST10_SENSOR_OP_OPEN_V", "ST10_START_OF_CLOSE_SENSOR_V", "ST10_SENSOR_OP_FULL_CLOSE_V", "ST10_RESPONSE_TIME_FWD", "ST10_RESPONSE_TIME_REV", "ST10_MOTOR_V_START_OF_CLOSE_A", "ST10_MOTOR_V_FULL_CLOSE_B", "ST10_MOTOR_V_START_BACK_C", "ST10_MOTOR_V_FULL_OPEN_D", "ST10_MOTOR_RMS_CURRENT_A", "ST10_FINAL_RST"], "table"="ST10_REPORT", "connection reference"=w1407) -> ("error out"=w1404:errorcluster, "connection reference out"=w1405:T16)  [unwired: 5 in]
              }
            }
            n520 = call <vilib>:"Simple Error Handler.vi"("type of dialog (OK msg:1)"=w1348, "error in (no error)"=w1349) -> ("error out"=w1347:errorcluster)  [unwired: 3 in, 4 out]
            n521 = call <vilib>:"Clear Errors.vi"("error in (no error)"=w1347) -> ("error out"=w1345:errorcluster)  [unwired: 5 in, 1 out]
            n522 = flat-sequence {
              tunnel: [w1357] -> w1335
              tunnel: w1345 -> [w1357]
              frame #0 {
                # "UPDATE op 20 save"
                n523 = global write "DATA LOG.vi" "OP 100 reset"(TRUE) -> ()
              }
            }
          }
          frame "DATALOG11" {
            (unwired) "WHERE BARCODE  ='%s'" ("format string")
            w1430 = T17 2 items=["no dialog", "OK message", "continue or stop message", "OK message + warnings", "continue/stop + warnings"] ("type of dialog (OK msg:1)")
            # "datalog of OP 110"
            n524 = call "PADMINI_AUTO_BARCODE_STRING 110.vi"("Enum"=enum16{"Read", "Write"}."Read", "error in (no error)"=w1421) -> ("error out"=w1420:errorcluster, "Input 2"=w1419:string[])  [unwired: 8 in]
            n525 = Index Array(array=w1419) -> (element=w1424:string)  [unwired: 1 in]
            n526 = call <vilib>:"Trim Whitespace.vi"("string"=w1424) -> ("trimmed string"=w1422:string)  [unwired: 1 in]
            n527 = call "String_Conversion_OP110.vi"("String in"=w1422) -> ("String out"=w1418:string)  [unwired: 9 in, 1 out]
            n528 = Index Array(array=w1419) -> (element #2=w1413:string, element #3=w1412:string)  [unwired: 3 in, 1 out]
            n529 = local read "SHIFT"() -> (w1409:string)
            n530 = call <vilib>:"Trim Whitespace.vi"("string"=w1412) -> ("trimmed string"=w1416:string)  [unwired: 1 in]
            n531 = call <vilib>:"Trim Whitespace.vi"("string"=w1413) -> ("trimmed string"=w1415:string)  [unwired: 1 in]
            n532 = call "PADMINI_SHIFT_DATE.vi"("SHIFT"=w1409) -> ("date/time string"=w1408:string)  [unwired: 10 in]
            n533 = Bundle("date/time string"=w1408, "trimmed string"=w1415, "trimmed string"=w1416) -> (w1411:T32)  [unwired: 1 in]
            n534 = Format Into String(format string="WHERE BARCODE  ='%s'", w1418) -> (resulting string=w1417:string)  [unwired: 2 in, 1 out]
            n535 = call <vilib>:"DB Tools Update Data.vi"("condition"=w1417, "data"=w1411, "error in (no error)"=w1420, "columns"=string[] ["OP110_DATE", "OP110_BIN_NO", "OP110_PALLET_NO"], "table"=w1434, "connection reference"=w1435) -> ("error out"=w1431:errorcluster, "connection reference out"=w1433:T16)  [unwired: 4 in]
            n536 = call <vilib>:"Simple Error Handler.vi"("type of dialog (OK msg:1)"=w1430, "error in (no error)"=w1431) -> ("error out"=w1429:errorcluster)  [unwired: 3 in, 4 out]
            n537 = call <vilib>:"Clear Errors.vi"("error in (no error)"=w1429) -> ("error out"=w1427:errorcluster)  [unwired: 5 in, 1 out]
            n538 = flat-sequence {
              tunnel: [w1438] -> w1425
              tunnel: w1427 -> [w1438]
              frame #0 {
                # "UPDATE op 20 save"
                n539 = global write "DATA LOG.vi" "OP 110 reset"(TRUE) -> ()
              }
            }
          }
          frame "EMERGENCY STOP" {
          }
          frame "STOP" {
            n540 = global read "Global 1.vi" "BARCODE RECIPE"() -> (w1449:string)
            n541 = Bundle("BARCODE RECIPE"=w1449) -> (w1448:cluster{"BARCODE RECIPE":string})  [unwired: 1 in]
            n542 = call <vilib>:"DB Tools Update Data.vi"("data"=w1448, "error in (no error)"=w1454, "columns"=string[] ["PREVIOUS_LOADED_RECIPE"], "table"="BARCODE_RECIPE", "connection reference"=w1452) -> ("error out"=w1453:errorcluster, "connection reference out"=w1451:T16)  [unwired: 5 in]
          }
        }
      }
      frame Error {
        # "Return true in any case that should stop the loop."
      }
    }
    n543 = Unbundle By Name(w131) -> ("OP - 90"=→"OP - 90":T33, "OP - 100"=→"OP - 100":T12, "OP - 110"=→"OP - 110":T9)
    n544 = Unbundle By Name(w131) -> ("OP - 10"=→"OP - 10":T34, "OP - 20"=→"OP - 20":T6, "OP - 30"=→"OP - 30":T35, "OP - 40"=→"OP - 40":T3)
    n545 = Unbundle By Name(w131) -> ("OP - 50"=→"OP - 50":T2, "OP - 60"=→"OP - 60":T36, "OP - 70"=→"OP - 70":T37, "OP - 80"=→"OP - 80":T38)
    n546 = Wait (ms)(milliseconds to wait=u32 100) -> ()  [unwired: 1 out]
    n547 = call <vilib>:"Simple Error Handler.vi"("error in (no error)"=w126) -> ("error out"=w125:errorcluster)  [unwired: 4 in, 4 out]
  }
  n548 = while {
    shift-right: [w1487] -> w73
    shift-left: w24 -> [w1481]
    shift-right: [w1488] -> w68
    shift-left: w71 -> [w1496]
    stop <- w1486 stop-if-true
    n549 = local read "Shift_change"() -> (w1494:bool)
    n550 = call <vilib>:"Clear Errors.vi"("error in (no error)"=w1481) -> ("error out"=w1472:errorcluster)  [unwired: 5 in, 1 out]
    n551 = call "READ EMERGENCY BIT.vi"("Enum"=enum16{"Read", "Write"}."Read", "error in (no error)"=w1472) -> ("Array Out"=w1484:dbl[])  [unwired: 8 in, 1 out]
    n552 = case shown="True" w1494 {
      tunnel: w1472 -> [w1513 w1526]
      tunnel: [w1514 w1525] -> w1493
      frame False {
        n553 = local read "SHIFT_DATA 2"() -> (w1516:string[])
        n554 = Get Date/Time In Seconds() -> (seconds since 1Jan1904=w1515:timestamp)
        n555 = call "String To Time_4.vi"("error in (no error)"=w1513, "String Array In"=w1516) -> ("error out"=w1512:errorcluster, "Time Stamp Out"=w1511:timestamp[])  [unwired: 8 in]
        "Time Stamp Out 4" <- w1511
        n556 = call "Shift Calculation_4.vi"("error in (no error)"=w1512, "Current Time"=w1515, "Time Stamp Out"=w1511) -> ("error out"=w1510:errorcluster, "Shift"=w1509:i32)  [unwired: 7 in]
        n557 = call <vilib>:"Clear Errors.vi"("error in (no error)"=w1510) -> ()  [unwired: 5 in, 2 out]
        n558 = case shown="4" w1509 {
          tunnel: ["A" "B" "C" "D"] -> w1514
          frame 1, Default {
          }
          frame 2 {
          }
          frame 3 {
          }
          frame 4 {
          }
        }
      }
      frame True {
        n559 = local read "SHIFT_DATA"() -> (w1524:string[])
        n560 = Get Date/Time In Seconds() -> (seconds since 1Jan1904=w1527:timestamp)
        n561 = call "String To Time.vi"("error in (no error)"=w1526, "String Array In"=w1524) -> ("error out"=w1523:errorcluster, "Time Stamp Out"=w1528:timestamp[])  [unwired: 8 in]
        "Time Stamp Out" <- w1528
        n562 = call "Shift Calculation.vi"("error in (no error)"=w1523, "Current Time"=w1527, "Time Stamp Out"=w1528) -> ("error out"=w1522:errorcluster, "Shift"=w1521:i32)  [unwired: 7 in]
        "Shift 4" <- w1521
        n563 = call <vilib>:"Clear Errors.vi"("error in (no error)"=w1522) -> ()  [unwired: 5 in, 2 out]
        n564 = case shown="3" w1521 {
          tunnel: ["A" "B" "C"] -> w1525
          frame 1, Default {
          }
          frame 2 {
          }
          frame 3 {
          }
        }
      }
    }
    "SHIFT" <- w1493
    n565 = Index Array(array=w1484) -> (element=w1483:dbl)  [unwired: 1 in]
    n566 = call "VALUE_CHANGE - ST1_RESULT.vi"("Numeric"=w1483) -> ("Boolean"=w1482:bool)  [unwired: 9 in, 1 out]
    n567 = global write "Global 1.vi" "EMERGENCY STOP"(w1482) -> ()
    n568 = call "Trigger_Loggic.vi"("error in (no error)"=w1472) -> ("error out"=w1477:errorcluster, "Array"=w1497:i32[])  [unwired: 9 in]
    n569 = global read "Global 1.vi" "PLC2 error"() -> (→"PLC2 error":errorcluster)
    n570 = global read "Global 1.vi" "PLC4 error"() -> (→"PLC4 error":errorcluster)
    n571 = global read "Global 1.vi" "PLC3 error"() -> (→"PLC3 error":errorcluster)
    n572 = global read "Global 1.vi" "PLC1 error"() -> (→"PLC1 error":errorcluster)
    n573 = for {
      tunnel: w1497 -> [w1532] mode=indexing
      shift-right: [w1536] -> w1490
      shift-left: w1496 -> [w1535]
      shift-right: [w1534] -> w1489
      shift-left: w1477 -> [w1533]
      n574 = case shown="2" w1532 {
        tunnel: [w1539 w1544 w1548 w1554 w1559 w1564 w1569 w1574 w1579 w1584 w1589 w1594 w1599 w1604 w1609 w1614 w1619 w1624 w1629 w1634 w1639 w1644 w1649] -> w1536
        tunnel: w1535 -> [w1541 w1546 w1549 w1556 w1561 w1566 w1571 w1576 w1581 w1586 w1591 w1596 w1601 w1606 w1611 w1616 w1621 w1626 w1631 w1636 w1641 w1646 w1651]
        tunnel: [w1538 w1543 w1550 w1553 w1558 w1563 w1568 w1573 w1578 w1583 w1588 w1593 w1598 w1603 w1608 w1613 w1618 w1623 w1628 w1633 w1638 w1643 w1648] -> w1534
        tunnel: w1533 -> [w1540 w1545 w1551 w1555 w1560 w1565 w1570 w1575 w1580 w1585 w1590 w1595 w1600 w1605 w1610 w1615 w1620 w1625 w1630 w1635 w1640 w1645 w1650]
        frame -1, Default {
          # "DEFAULT"
          n575 = Enqueue Element(queue=w1541, element=cluster{"CASE 2":T15} {"CASE 2"=enum."-1"}, error in (no error)=w1540) -> (queue out=w1539:refnum<queue>, error out=w1538:errorcluster)  [unwired: 1 in, 1 out]
        }
        frame 0 {
          # "SCAN BARCODE OP 10"
          n576 = Enqueue Element(queue=w1546, element=cluster{"CASE 2":T15} {"CASE 2"=enum."-1"}, error in (no error)=w1545) -> (queue out=w1544:refnum<queue>, error out=w1543:errorcluster)  [unwired: 1 in, 1 out]
        }
        frame 1 {
          # "DATALOG OF OP 10"
          n577 = Enqueue Element(queue=w1549, element=cluster{"CASE 2":T15} {"CASE 2"=enum."SCAN1"}, error in (no error)=w1551) -> (queue out=w1548:refnum<queue>, error out=w1550:errorcluster)  [unwired: 1 in, 1 out]
        }
        frame 2 {
          # "SCAN BARCODE OP 20"
          n578 = Enqueue Element(queue=w1556, element=cluster{"CASE 2":T15} {"CASE 2"=enum."SCAN2"}, error in (no error)=w1555) -> (queue out=w1554:refnum<queue>, error out=w1553:errorcluster)  [unwired: 1 in, 1 out]
        }
        frame 3 {
          # "DATALOG OF OP 20"
          n579 = Enqueue Element(queue=w1561, element=cluster{"CASE 2":T15} {"CASE 2"=enum."DATALOG2"}, error in (no error)=w1560) -> (queue out=w1559:refnum<queue>, error out=w1558:errorcluster)  [unwired: 1 in, 1 out]
        }
        frame 4 {
          # "SCAN BARCODE OP 30"
          n580 = Enqueue Element(queue=w1566, element=cluster{"CASE 2":T15} {"CASE 2"=enum."SCAN3"}, error in (no error)=w1565) -> (queue out=w1564:refnum<queue>, error out=w1563:errorcluster)  [unwired: 1 in, 1 out]
        }
        frame 5 {
          # "DATALOG OF OP 30"
          n581 = Enqueue Element(queue=w1571, element=cluster{"CASE 2":T15} {"CASE 2"=enum."DATALOG3"}, error in (no error)=w1570) -> (queue out=w1569:refnum<queue>, error out=w1568:errorcluster)  [unwired: 1 in, 1 out]
        }
        frame 6 {
          # "SCAN BARCODE OP 40"
          n582 = Enqueue Element(queue=w1576, element=cluster{"CASE 2":T15} {"CASE 2"=enum."SCAN4"}, error in (no error)=w1575) -> (queue out=w1574:refnum<queue>, error out=w1573:errorcluster)  [unwired: 1 in, 1 out]
        }
        frame 7 {
          # "DATALOG OF OP 40"
          n583 = Enqueue Element(queue=w1581, element=cluster{"CASE 2":T15} {"CASE 2"=enum."DATALOG4"}, error in (no error)=w1580) -> (queue out=w1579:refnum<queue>, error out=w1578:errorcluster)  [unwired: 1 in, 1 out]
        }
        frame 8 {
          # "SCAN BARCODE OP 50"
          n584 = Enqueue Element(queue=w1586, element=cluster{"CASE":T15} {"CASE"=enum."SCAN5"}, error in (no error)=w1585) -> (queue out=w1584:refnum<queue>, error out=w1583:errorcluster)  [unwired: 1 in, 1 out]
        }
        frame 9 {
          # "DATALOG OF OP 50"
          n585 = Enqueue Element(queue=w1591, element=cluster{"CASE":T15} {"CASE"=enum."DATALOG5"}, error in (no error)=w1590) -> (queue out=w1589:refnum<queue>, error out=w1588:errorcluster)  [unwired: 1 in, 1 out]
        }
        frame 10 {
          # "SCAN BARCODE OP 60"
          n586 = Enqueue Element(queue=w1596, element=cluster{"CASE 2":T15} {"CASE 2"=enum."SCAN6"}, error in (no error)=w1595) -> (queue out=w1594:refnum<queue>, error out=w1593:errorcluster)  [unwired: 1 in, 1 out]
        }
        frame 11 {
          # "DATALOG OF OP 60"
          n587 = Enqueue Element(queue=w1601, element=cluster{"CASE 2":T15} {"CASE 2"=enum."DATALOG6"}, error in (no error)=w1600) -> (queue out=w1599:refnum<queue>, error out=w1598:errorcluster)  [unwired: 1 in, 1 out]
        }
        frame 12 {
          # "SCAN BARCODE OP 70"
          n588 = Enqueue Element(queue=w1606, element=cluster{"CASE 2":T15} {"CASE 2"=enum."SCAN7"}, error in (no error)=w1605) -> (queue out=w1604:refnum<queue>, error out=w1603:errorcluster)  [unwired: 1 in, 1 out]
        }
        frame 13 {
          # "DATALOG OF OP 70"
          n589 = Enqueue Element(queue=w1611, element=cluster{"CASE 2":T15} {"CASE 2"=enum."DATALOG7"}, error in (no error)=w1610) -> (queue out=w1609:refnum<queue>, error out=w1608:errorcluster)  [unwired: 1 in, 1 out]
        }
        frame 14 {
          # "SCAN BARCODE 80"
          n590 = Enqueue Element(queue=w1616, element=cluster{"CASE 2":T15} {"CASE 2"=enum."SCAN8"}, error in (no error)=w1615) -> (queue out=w1614:refnum<queue>, error out=w1613:errorcluster)  [unwired: 1 in, 1 out]
        }
        frame 15 {
          # "DATALOG OF OP 80"
          n591 = Enqueue Element(queue=w1621, element=cluster{"CASE 2":T15} {"CASE 2"=enum."DATALOG8"}, error in (no error)=w1620) -> (queue out=w1619:refnum<queue>, error out=w1618:errorcluster)  [unwired: 1 in, 1 out]
        }
        frame 16 {
          # "SCAN BARCODE OP 90"
          n592 = Enqueue Element(queue=w1626, element=cluster{"CASE 2":T15} {"CASE 2"=enum."SCAN9"}, error in (no error)=w1625) -> (queue out=w1624:refnum<queue>, error out=w1623:errorcluster)  [unwired: 1 in, 1 out]
        }
        frame 17 {
          # "DATALOG OF OP 90"
          n593 = Enqueue Element(queue=w1631, element=cluster{"CASE 2":T15} {"CASE 2"=enum."DATALOG9"}, error in (no error)=w1630) -> (queue out=w1629:refnum<queue>, error out=w1628:errorcluster)  [unwired: 1 in, 1 out]
        }
        frame 18 {
          # "SCAN BARCODE OP 100"
          n594 = Enqueue Element(queue=w1636, element=cluster{"CASE 2":T15} {"CASE 2"=enum."SCAN10"}, error in (no error)=w1635) -> (queue out=w1634:refnum<queue>, error out=w1633:errorcluster)  [unwired: 1 in, 1 out]
        }
        frame 19 {
          # "DATALOG OF OP 100"
          n595 = Enqueue Element(queue=w1641, element=cluster{"CASE 2":T15} {"CASE 2"=enum."DATALOG10"}, error in (no error)=w1640) -> (queue out=w1639:refnum<queue>, error out=w1638:errorcluster)  [unwired: 1 in, 1 out]
        }
        frame 20 {
          # "SCAN BARCODE OP 110"
          n596 = Enqueue Element(queue=w1646, element=cluster{"CASE 2":T15} {"CASE 2"=enum."SCAN11"}, error in (no error)=w1645) -> (queue out=w1644:refnum<queue>, error out=w1643:errorcluster)  [unwired: 1 in, 1 out]
        }
        frame 21 {
          # "DATALOG OF OP 110"
          n597 = Enqueue Element(queue=w1651, element=cluster{"CASE 2":T15} {"CASE 2"=enum."DATALOG11"}, error in (no error)=w1650) -> (queue out=w1649:refnum<queue>, error out=w1648:errorcluster)  [unwired: 1 in, 1 out]
        }
      }
    }
    n598 = global read "Global 1.vi" "PLC5 error"() -> (→"PLC5 error":errorcluster)
    n599 = global read "Global 1.vi" "PLC6 error"() -> (→"PLC6 error":errorcluster)
    n600 = global read "Global 1.vi" "PLC7 error"() -> (→"PLC7 error":errorcluster)
    n601 = global read "Global 1.vi" "PLC8 error"() -> (→"PLC8 error":errorcluster)
    n602 = Wait (ms)(milliseconds to wait=u32 50) -> ()  [unwired: 1 out]
    n603 = global read "Global 1.vi" "PLC COMM"() -> (→"PLC COM.":bool)
    n604 = global read "Global 1.vi" "PLC 1"() -> (→"OP 10 & 20":bool)
    n605 = global read "Global 1.vi" "PLC 2"() -> (→"OP 30":bool)
    n606 = global read "Global 1.vi" "PLC 3"() -> (→"OP 40":bool)
    n607 = case shown="True" "stop 2" {
      tunnel: w1490 -> [w1500 w1506]
      tunnel: [w1500 w1505] -> w1488
      tunnel: w1489 -> [w1499 w1504]
      tunnel: [w1499 w1503] -> w1487
      tunnel: [FALSE TRUE] -> w1486
      frame False {
      }
      frame True {
        n608 = Flush Queue(queue=w1506, error in (no error)=w1504) -> (queue out=w1508:refnum<queue>, error out=w1507:errorcluster)  [unwired: 1 out]
        n609 = Enqueue Element(queue=w1508, element=cluster{"CASE 2":T15} {"CASE 2"=enum."STOP"}, error in (no error)=w1507) -> (queue out=w1505:refnum<queue>, error out=w1503:errorcluster)  [unwired: 1 in, 1 out]
      }
    }
    "stop" <- w1486
    n610 = global read "Global 1.vi" "PLC 4"() -> (→"OP 50":bool)
    n611 = global read "Global 1.vi" "PLC 5"() -> (→"OP 60":bool)
    n612 = global read "Global 1.vi" "PLC 6"() -> (→"OP 70 & 80":bool)
    n613 = global read "Global 1.vi" "PLC 7"() -> (→"OP 90 -100":bool)
    n614 = global read "Global 1.vi" "PLC 8"() -> (→"OP 110":bool)
  }
  n615 = Release Queue(queue=w68, error in (no error)=w73) -> (error out=w51:errorcluster)  [unwired: 1 in, 2 out]
  n616 = call <vilib>:"Clear Errors.vi"("error in (no error)"=w69) -> ("error out"=w55:errorcluster)  [unwired: 5 in, 1 out]
  n617 = Not A Number/Path/Refnum?(number/path/refnum=w2) -> (NaN/Path/Refnum?=w1:bool)
  n618 = case shown="True" w1 {
    tunnel: w55 -> [w1654 w1655]
    tunnel: [w1653 w1655] -> w52
    tunnel: w2 -> [w1652 _]
    frame False {
      n619 = call <vilib>:"DB Tools Close Connection.vi"("error in (no error)"=w1654, "connection reference"=w1652) -> ("error out"=w1653:errorcluster)  [unwired: 5 in]
    }
    frame True {
    }
  }
  n620 = Merge Errors(w51, w52) -> (w53:errorcluster)
  n621 = call <vilib>:"Simple Error Handler.vi"("error in (no error)"=w53) -> ("error out"=w48:errorcluster)  [unwired: 4 in, 4 out]
  n622 = call <vilib>:"Clear Errors.vi"("error in (no error)"=w48) -> ("error out"=w54:errorcluster)  [unwired: 5 in, 1 out]
  n623 = flat-sequence {
    tunnel: w54 -> [w1658]
    tunnel: [w1658] -> w56
    frame #0 {
      n624 = global write "Global 1.vi" "REMOVE VI"(TRUE ("remove_VI")) -> ()
      n625 = global write "DATA LOG.vi" "Auto Cycle On"(FALSE) -> ()
    }
  }
  n626 = property class="App"(error in=w56) -> (error out=w58:errorcluster, "App.Kind"=w57:T39)  [unwired: 1 in, 1 out]
  n627 = case shown="\"Run Time System\"" w57 {
    tunnel: [w1659 w1661] -> w59
    tunnel: w58 -> [w1659 w1660]
    frame "Development System", Default {
    }
    frame "Run Time System" {
      n628 = invoke class="VI" method="FP.Close"(error in=w1660) -> (error out=w1661:errorcluster)  [unwired: 2 in, 2 out]
    }
  }
  "error out 2" <- w59
